vi "Autonomous Independent.vi"() -> ()   [LabVIEW 2017]
doc: "This VI is called when autonomous begins, and will automatically be terminated when autonomous ends. You can carry out timed or sensor driven robot movement independently without needing to return to the caller."
uses:
  Public/Documents/Cross The Road Electronics/Phoenix-LabVIEW/Motor Controller/Controls/CTRE_Phoenix_MotorControl_ControlMode.ctl
  <vilib>/Rock Robotics/WPI/DriverStation/WPI_DriverStationAllianceInfo.ctl
  <vilib>/Rock Robotics/WPI/Relay/WPI_RelayValue.ctl
  <vilib>/Rock Robotics/WPI/SerialPort/WPI_SerialPort.ctl
  <vilib>/Rock Robotics/WPI/Utilities/WPI_GetSetVariantRefNum.vi
  Public/Documents/Cross The Road Electronics/Phoenix-LabVIEW/Motor Controller/Get/CTRE_Phoenix_MotorController_GetPulseWidthAll.vi
  Robot Global Data.vi
  <vilib>/Utility/config.llb/Read Key (Double).vi
  Public/Documents/Cross The Road Electronics/Phoenix-LabVIEW/Motor Controller/Get/CTRE_Phoenix_MotorController_GetSelectedSensorData.vi
  Public/Documents/Cross The Road Electronics/Phoenix-LabVIEW/Motor Controller/Get/CTRE_Phoenix_MotorController_GetQuadratureData.vi
  <vilib>/Rock Robotics/WPI/Solenoid/Deprecated/WPI_SolenoidSetBool.vi
  <vilib>/Utility/config.llb/NI_LVConfig.lvlib
panel:
  out "Current Pos 3":dbl
  out "Current Pos 2":dbl
  out "Current Pos 1":dbl
  out "Current Pos 0":dbl
  out "ElevatorScale":dbl
  out "ElevatorSwitch":dbl
  out "ElevatorPyramid":dbl
  out "ElevatorDown":dbl
  out "ElevatePos":dbl
  out "CoolDown":bool
  out "MidSwitchPosition":dbl
  out "zChange":dbl
  out "Gyro":dbl
  out "Zero Gyro":bool
  out "Autonomous Select":dbl
  out "Direction":dbl
  out "stopped":bool
  out "speed":dbl
  out "Direction 3":dbl
  out "Direction 2":dbl
  out "Direction 1":dbl
  out "x":dbl
  out "Current Reading":string
  out "Text":string
  out "Switch":bool
  out "Scale":bool
  out "Rel Pos 3":i32
  out "Rel Pos 2":i32
  out "Rel Pos 1":i32
  out "Rel Pos 0":i32
  out "Final Rel Pos 3":i32
  out "Final Rel Pos 2":i32
  out "Final Rel Pos 1":i32
  out "Final Rel Pos 0":i32
  out "Start Pos 3":i32
  out "Start Pos 2":i32
  out "Start Pos 1":i32
  out "Start Pos 0":i32
  # "Be sure to right-click and choose Data Operations>>Make Current Value default if you want to save the array values with the VI"
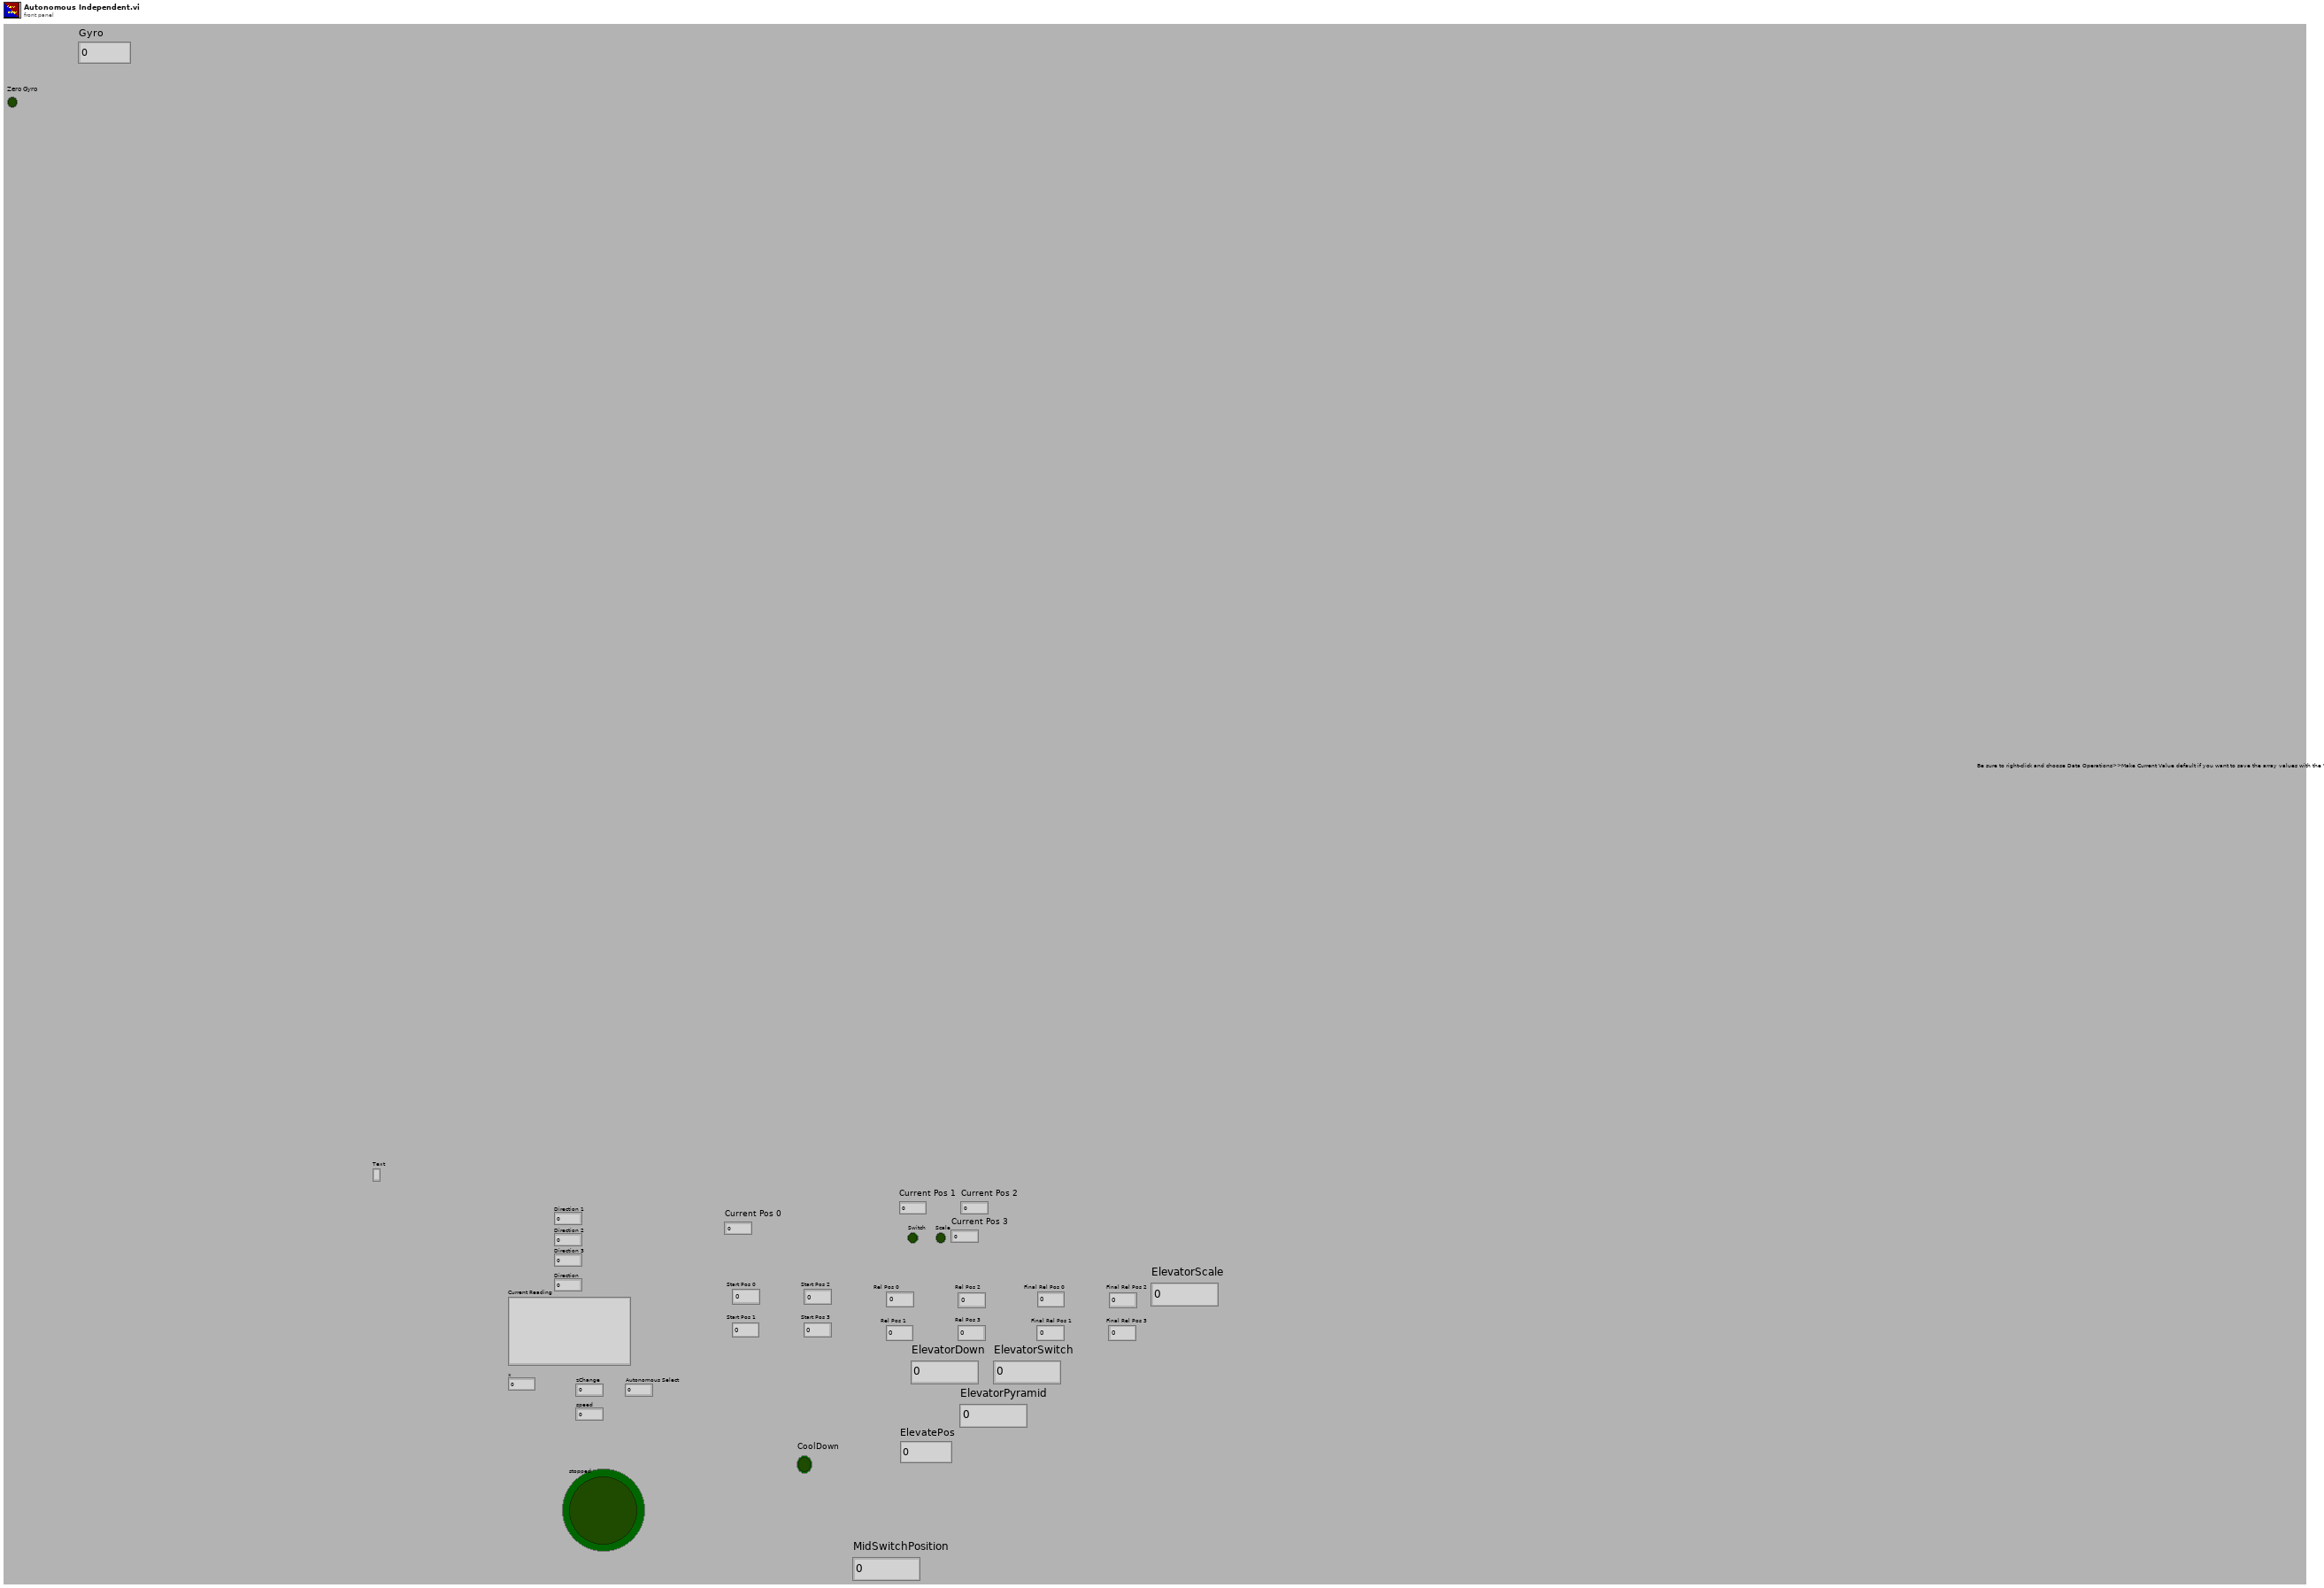
[diagram p1: front panel]
types:
  T1 = typedef "WPI_JoystickDevRef.ctl" = cluster{"Device":T2}
  T2 = typedef "WPI_JoystickDeviceEnum.ctl" = enum16{"USB 0", "USB 1", "USB 2", "USB 3", "USB 4", "USB 5"}
  T3 = typedef "WPI_DriverStationAllianceInfo.ctl" = enum16{"Red", "Blue", "Invalid"}
  T4 = typedef "WPI_RelayValue.ctl" = enum16{"Off", "On", "Forward", "Reverse"}
  T5 = typedef "WPI_SerialPort.ctl" = enum16{"Onboard RS-232", "MXP TTL", "USB 1", "USB 2"}
  T6 = typedef "CTRE_Phoenix_MotorControl_ControlMode.ctl" = u16
  T7 = typedef "WPI_GyroDevRef.ctl" = cluster{"DevStatus":errorcluster, "Analog Channel":T8, "Gain (VoltsPerDegree/Second)":dbl, "Gyro Type":enum16{"Analog", "XRS450"}, "Handle":i32, "SPI Bus":T9, "Device Found":bool, "Sample Rate":dbl, "Calibrate On Open":bool, "Offset":dbl}
  T8 = typedef "FPGA_AIChannel.ctl" = enum8{"AI 0", "AI 1", "AI 2", "AI 3", "AI MXP 0", "AI MXP 1", "AI MXP 2", "AI MXP 3", "Invalid"}
  T9 = typedef "spi_bus.ctl" = enum16{"SPI On-Board, CS0", "SPI On-Board, CS1", "SPI On-Board, CS2", "SPI On-Board, CS3", "SPI MXP", "Invalid"}
  T10 = typedef "WPI_MotorControlDeviceRef.ctl" = cluster{"DeviceStatus":errorcluster, "Type":T11, "PWM":cluster{"PWM Channel":T12, "DeadBand":T13}, "CAN":cluster{"Device Number":u8, "SetOutput VI Ref":variant, "GetOutput VI Ref":variant, "Enable VI Ref":variant, "Disable VI Ref":variant, "Data":variant}, "Invert":bool, "DIO PWM":cluster{"PWM \"Enable\" Channel":T12, "DIOChannel":T14, "PWM Rate":dbl}}
  T11 = typedef "WPI_MotorControlType.ctl" = enum16{"PWM", "CAN", "DIO PWM"}
  T12 = typedef "FPGA_DIOPWMChannel.ctl" = enum8{"PWM 0", "PWM 1", "PWM 2", "PWM 3", "PWM 4", "PWM 5", "PWM 6", "PWM 7", "PWM 8", "PWM 9", "PWM MXP 0", "PWM MXP 1", "PWM MXP 2", "PWM MXP 3", "PWM MXP 4", "PWM MXP 5", "PWM MXP 6", "PWM MXP 7", "PWM MXP 8", "PWM MXP 9", "Invalid"}
  T13 = typedef "WPI_PWMDeadband.ctl" = cluster{"Name":string, "maxPositivePwm":i32, "minPositivePwm":i32, "centerPwm":i32, "maxNegativePwm":i32, "minNegativePwm":i32, "angularRange":u16}
  T14 = typedef "FPGA_DIOChannel.ctl" = enum8{"DIO 0", "DIO 1", "DIO 2", "DIO 3", "DIO 4", "DIO 5", "DIO 6", "DIO 7", "DIO 8", "DIO 9", "DIO MXP 0", "DIO MXP 1", "DIO MXP 2", "DIO MXP 3", "DIO MXP 4", "DIO MXP 5", "DIO MXP 6", "DIO MXP 7", "DIO MXP 8", "DIO MXP 9", "DIO MXP 10", "DIO MXP 11", "DIO MXP 12", "DIO MXP 13", "DIO MXP 14", "DIO MXP 15", "SPI Port CS1", "SPI Port CS2", "SPI Port CS3", "SPI Port MISO", "SPI Port MOSI", "Invalid"}
  T15 = typedef "NI_LVConfig.lvlib/Config Data RefNum.ctl" = refnum<k1>
  T16 = typedef "WPI_RelayDevRef.ctl" = cluster{"DevStatus":errorcluster, "Relay Channel":T17, "Relay Direction":T18}
  T17 = typedef "FPGA_DIORelayChannel.ctl" = enum8{"Relay 0", "Relay 1", "Relay 2", "Relay 3", "Invalid"}
  T18 = typedef "WPI_RelayDirection.ctl" = enum16{"Both directions", "Forward only", "Reverse only"}
  T19 = typedef "WPI_SerialPortRef.ctl" = cluster{"DevStatus":errorcluster, "Serial Port Name":refnum<visa-resource-name>}
  T20 = typedef "WPI_SolenoidDevRef.ctl" = cluster{"DevStatus":errorcluster, "Pneumatics Control Module":u8, "Forward Solenoid Channel":T21, "Reverse Solenoid Channel":T21}
  T21 = typedef "WPI_SolenoidChannel.ctl" = enum8{"Solenoid 0", "Solenoid 1", "Solenoid 2", "Solenoid 3", "Solenoid 4", "Solenoid 5", "Solenoid 6", "Solenoid 7", "Invalid"}
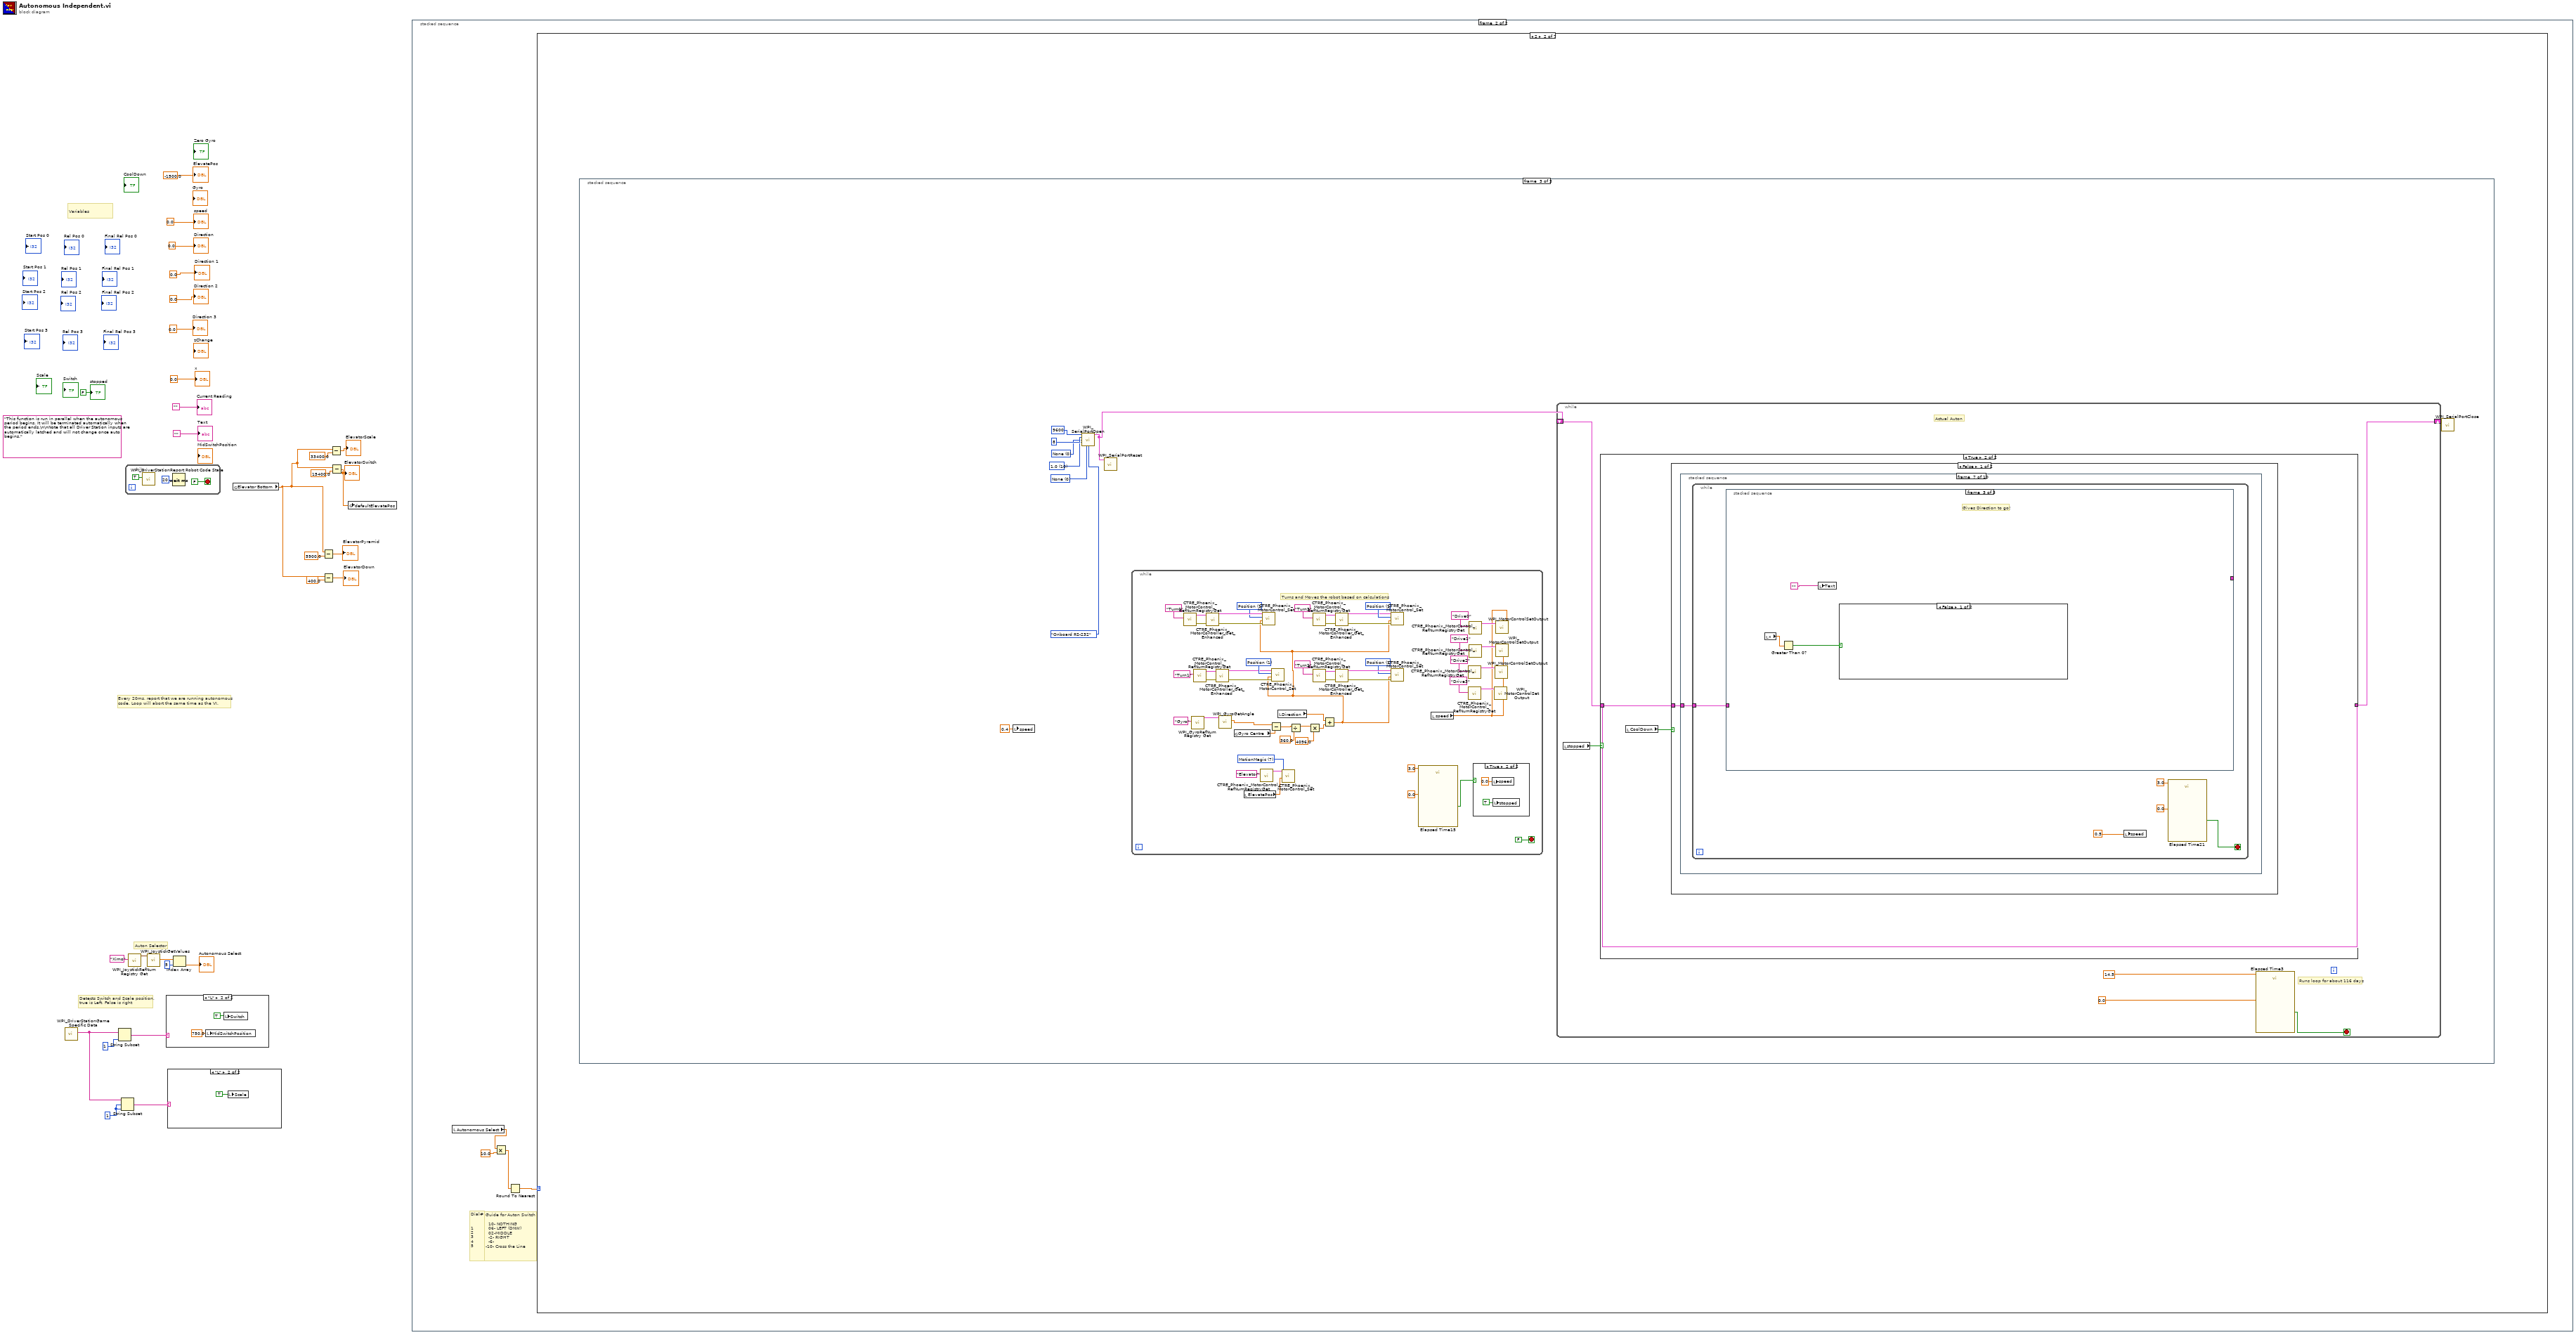
[diagram p0: block diagram]
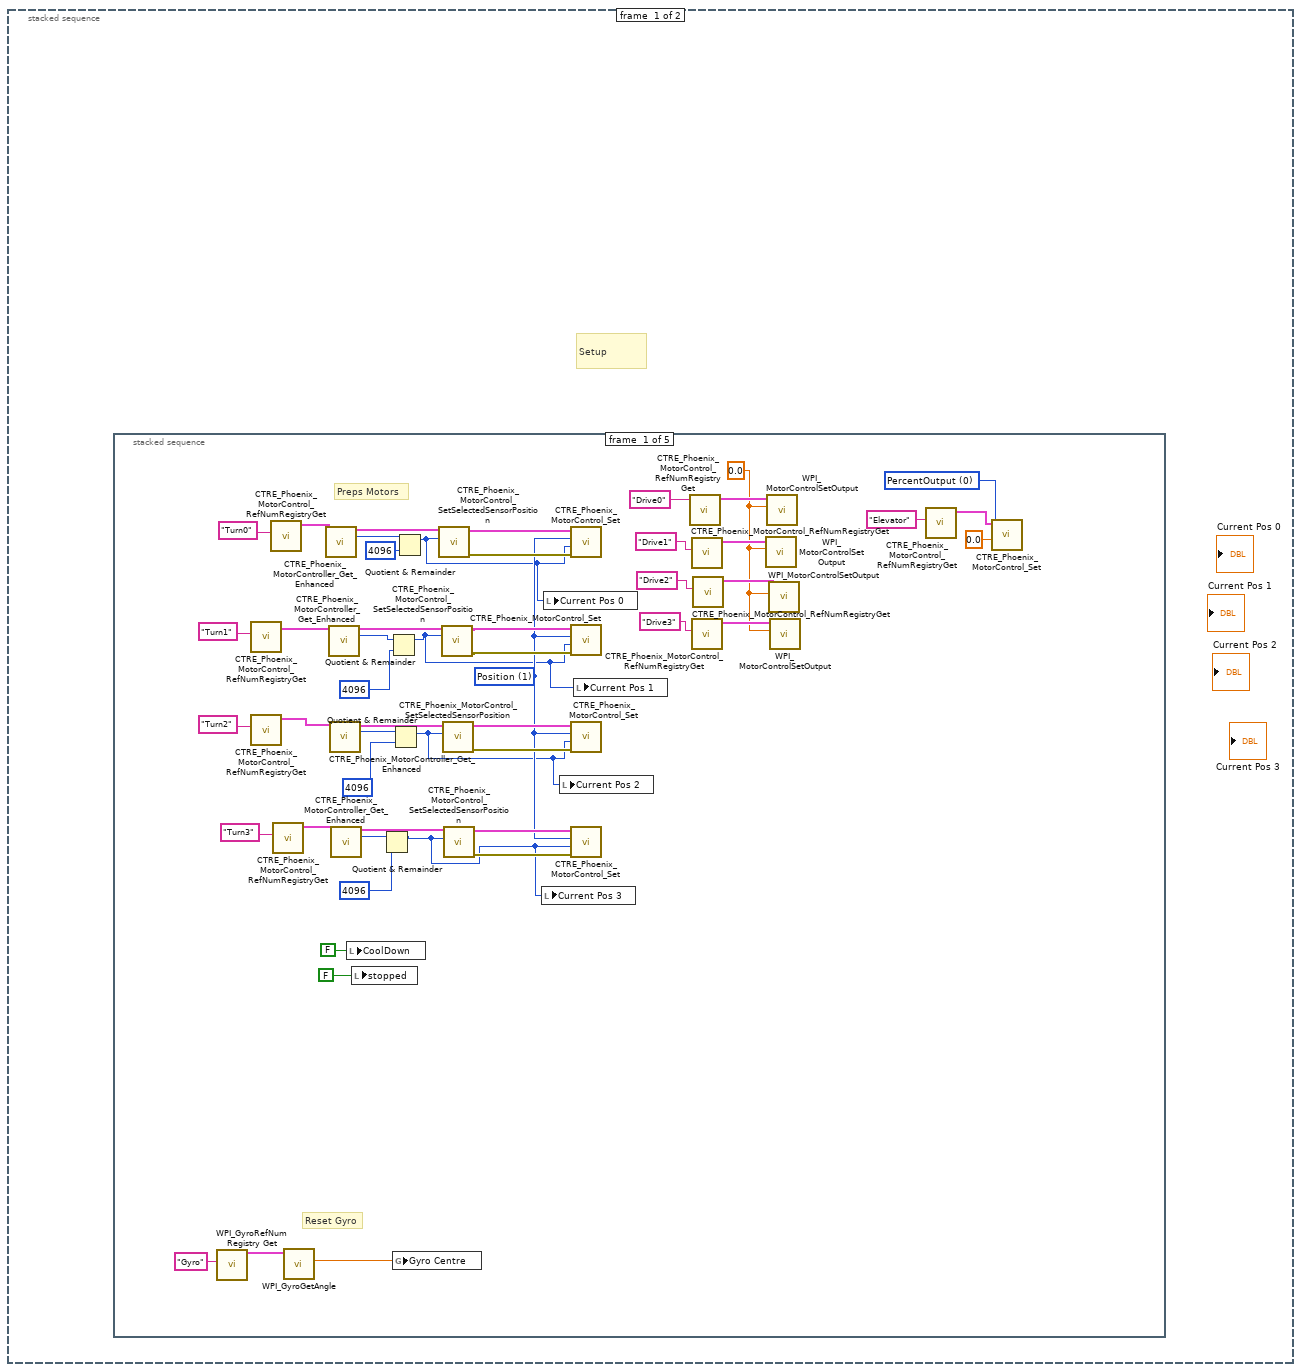
[diagram p2: hidden frame]
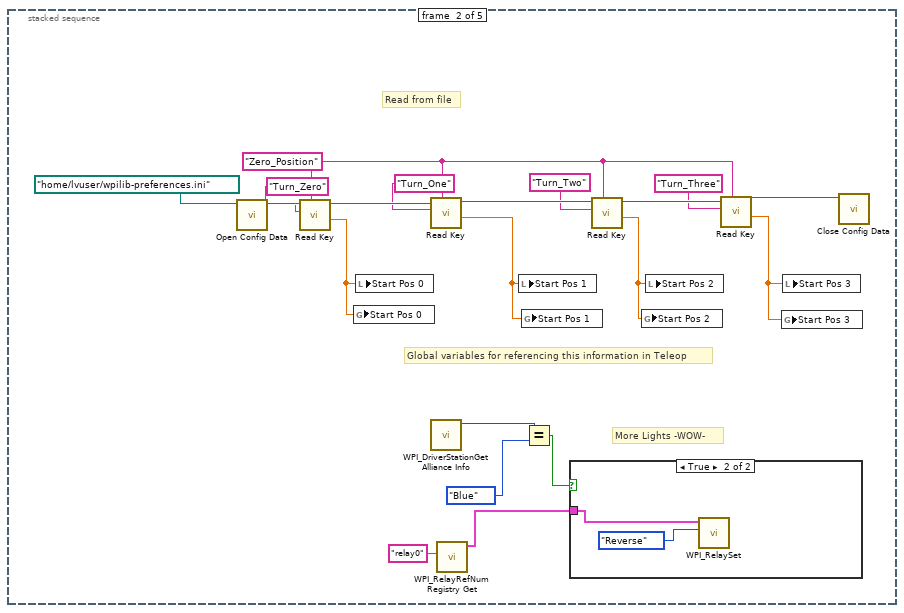
[diagram p3: hidden frame]
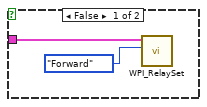
[diagram p4: hidden frame]
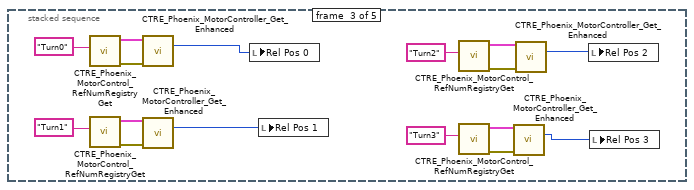
[diagram p5: hidden frame]
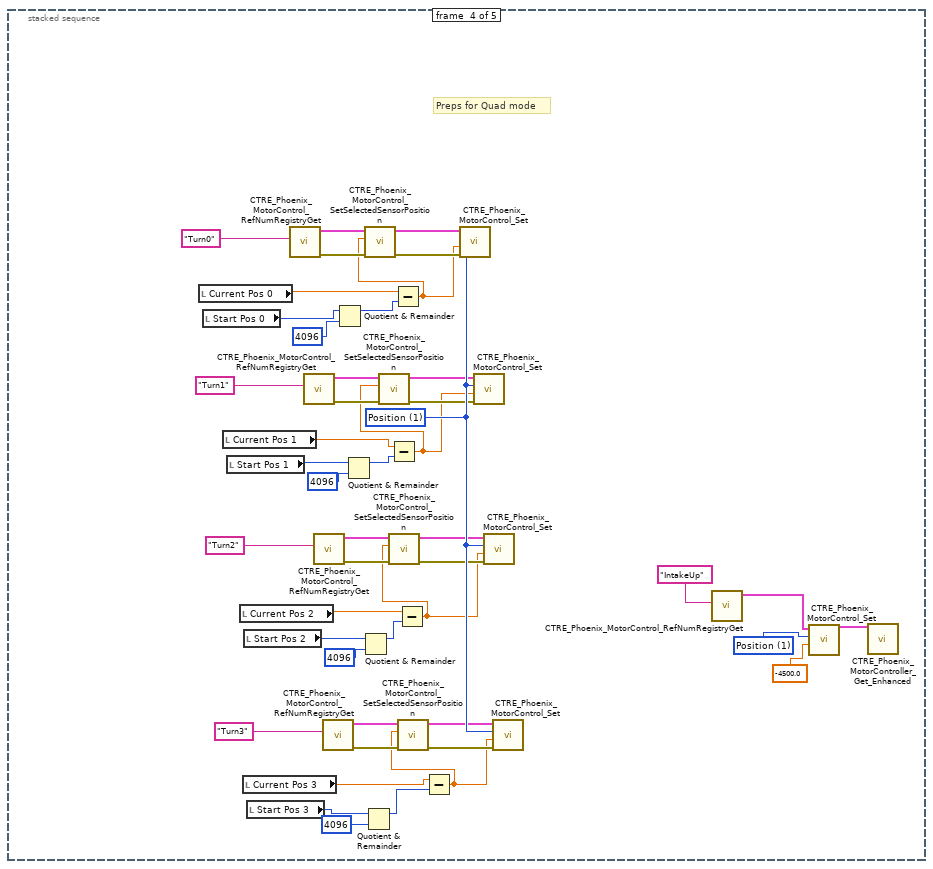
[diagram p6: hidden frame]
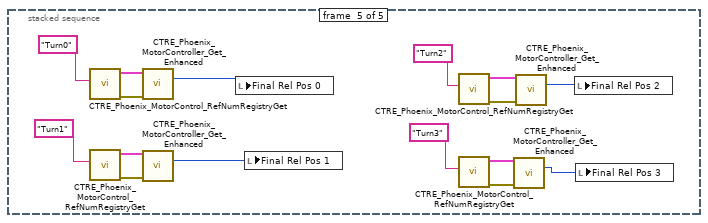
[diagram p7: hidden frame]
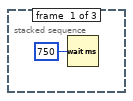
[diagram p9: hidden frame]
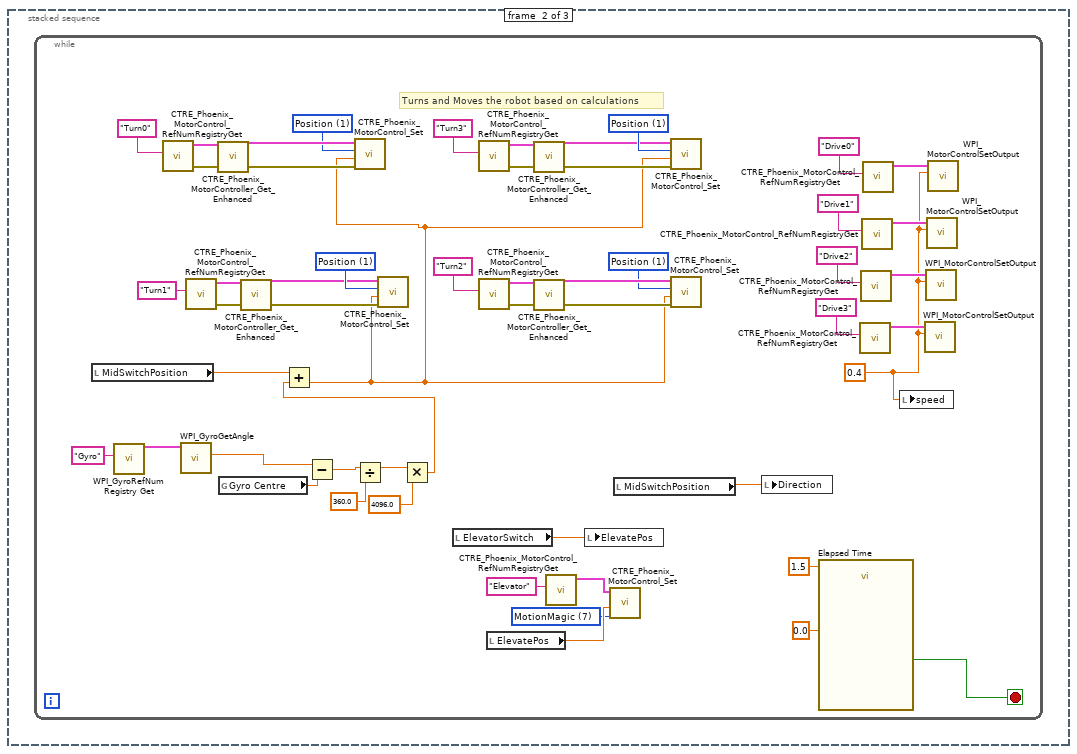
[diagram p10: hidden frame]
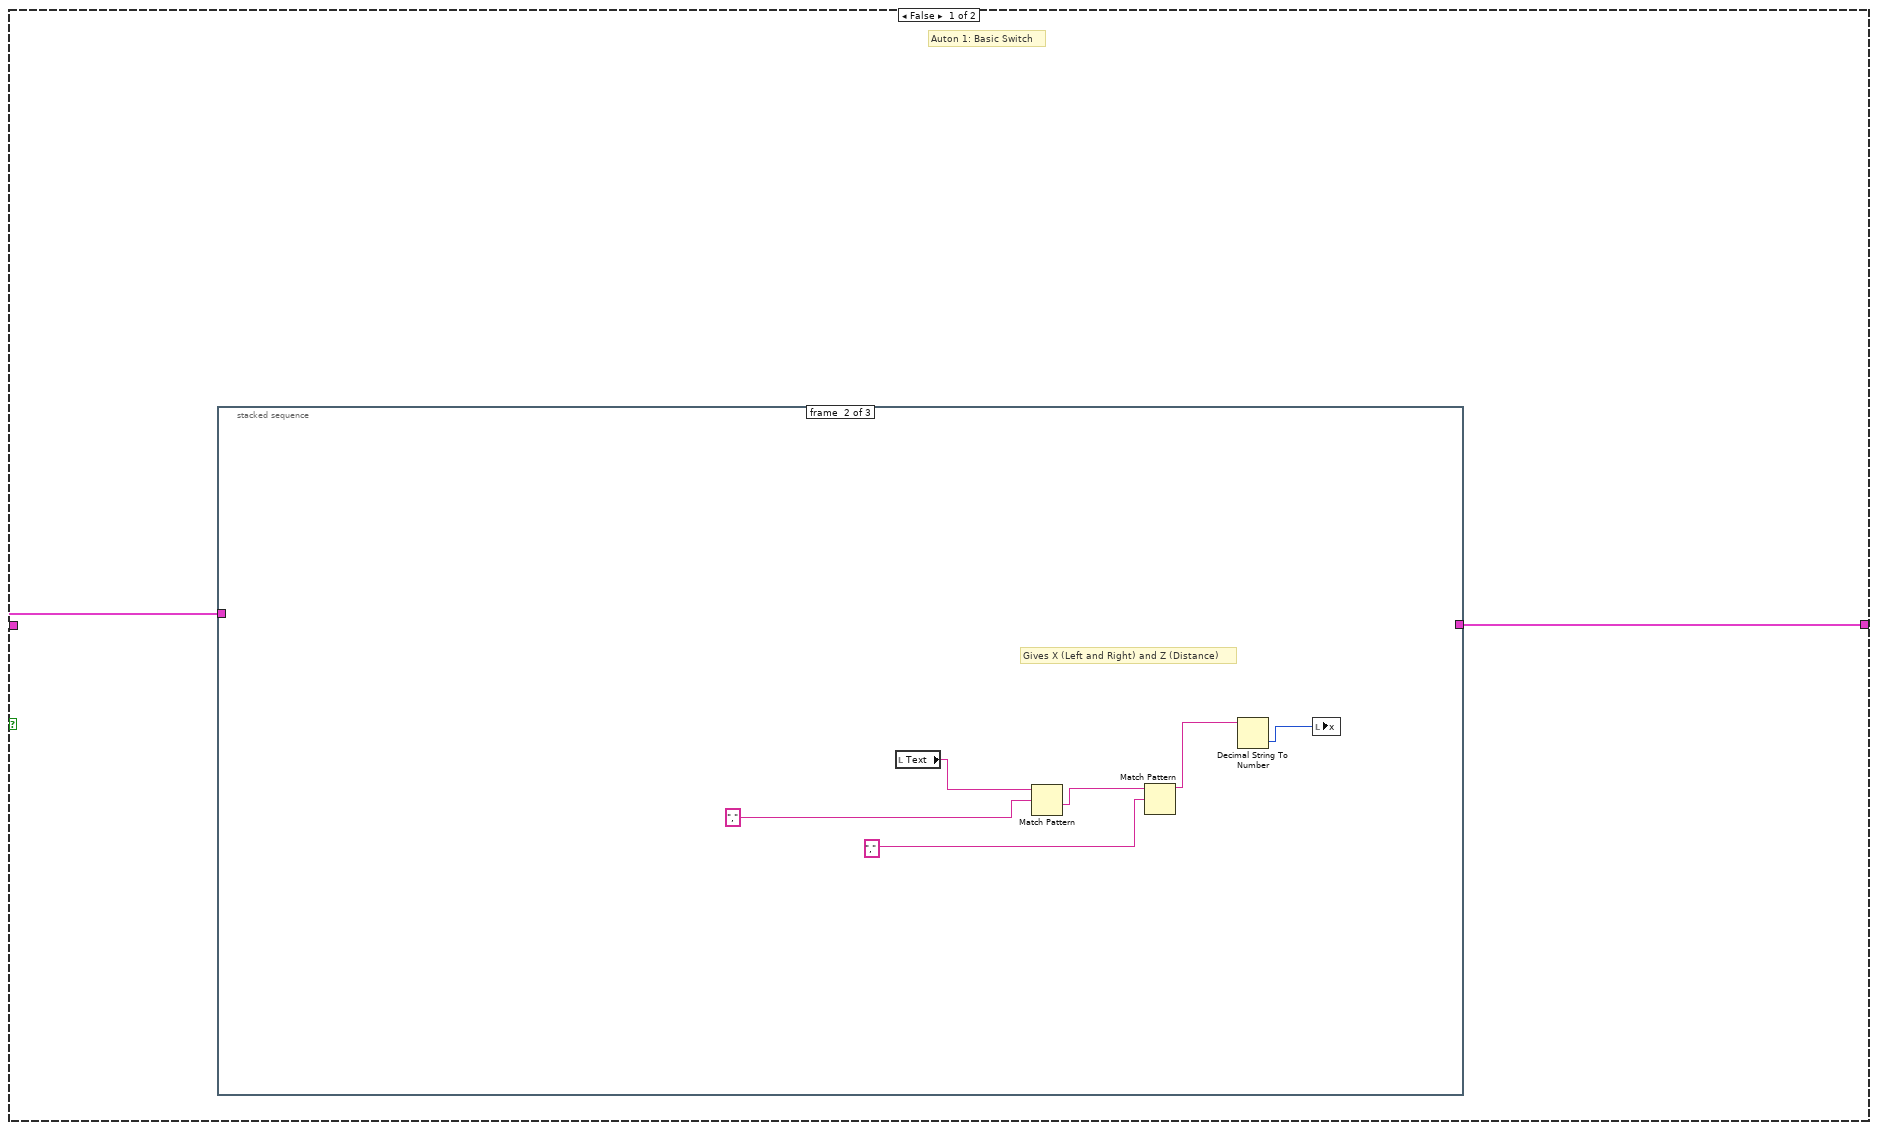
[diagram p12: hidden frame]
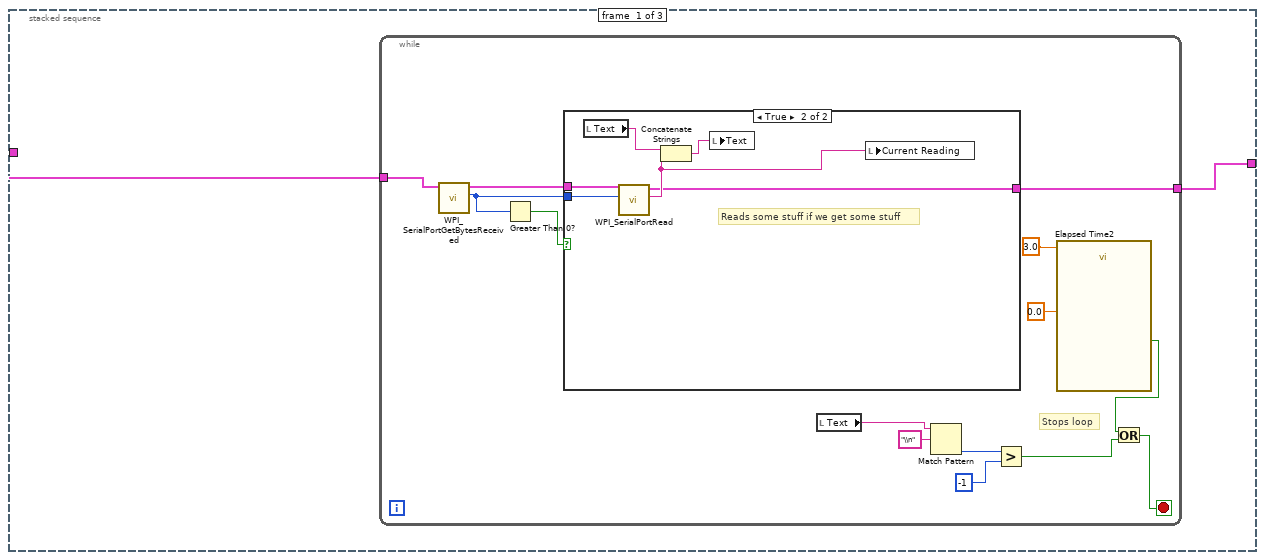
[diagram p13: hidden frame]
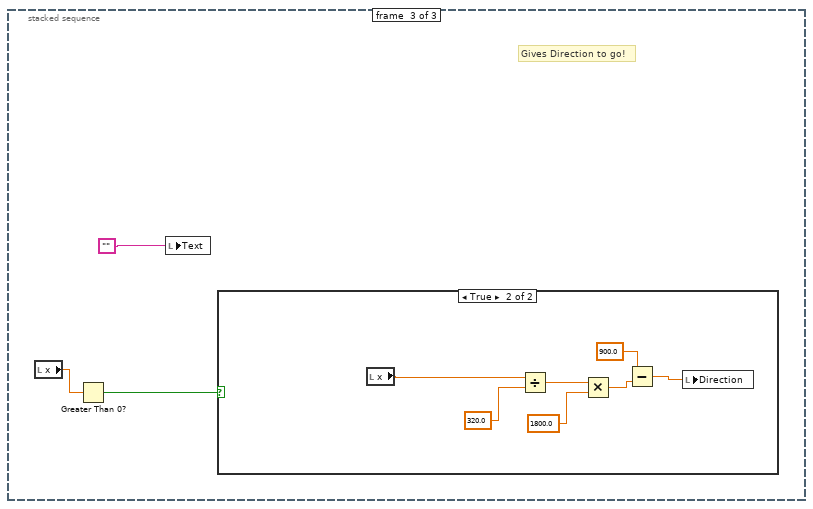
[diagram p15: hidden frame]
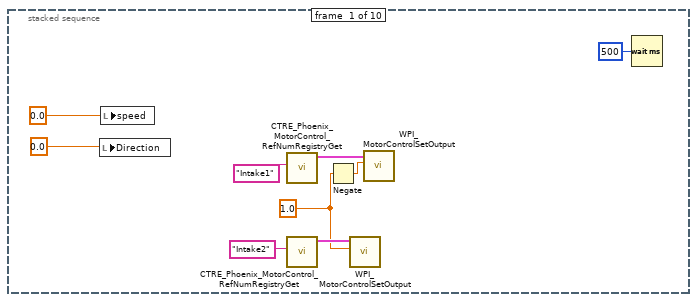
[diagram p17: hidden frame]
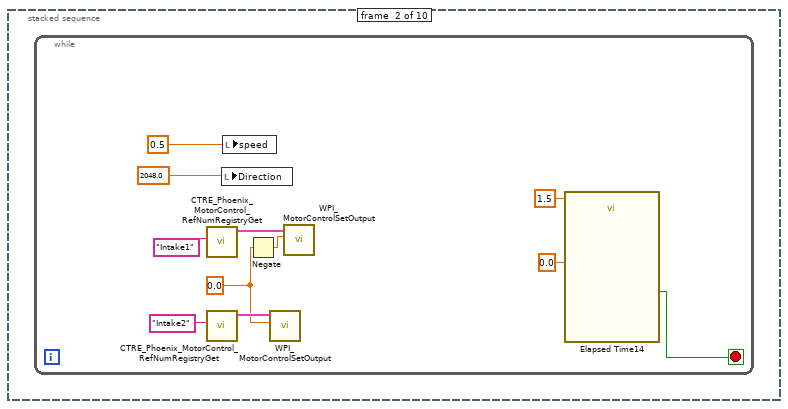
[diagram p18: hidden frame]
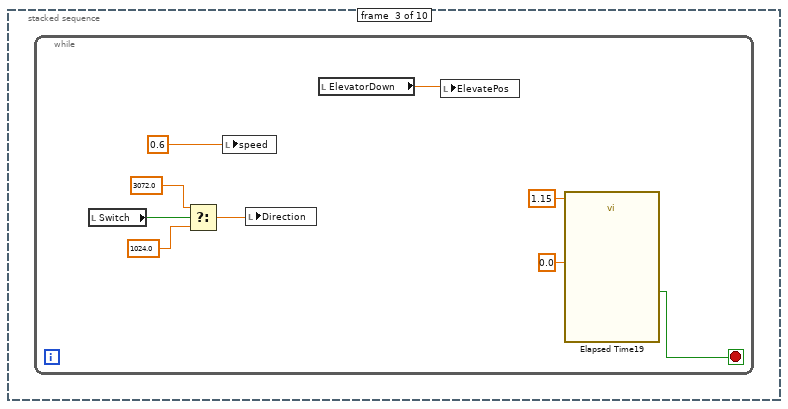
[diagram p19: hidden frame]
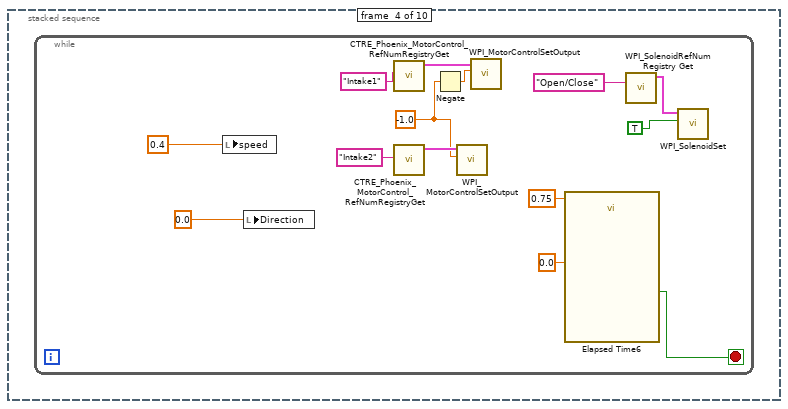
[diagram p20: hidden frame]
diagram:
  w26 = 1 ("length (rest)")
  (unwired) "This function is run in parallel when the autonomous period begins. It will be terminated automatically when the period ends.\n\nNote that all Driver Station inputs are automatically latched and will not change once auto begins."
  # "Auton Selector"
  # "Variables"
  # "Detects Switch and Scale position,\ntrue is Left, False is right"
  # "Every 20ms, report that we are running autonomous\ncode. Loop will abort the same time as the VI."
  n1 = call <vilib>:"WPI_DriverStationGame Specific Data.vi"() -> ("Game Specific Data"=w25:string)  [unwired: 11 in]
  n2 = String Subset(string=w25, length (rest)=1 ("length (rest)")) -> (substring=w29:string)  [unwired: 1 in]
  n3 = String Subset(string=w25, offset (0)=w26, length (rest)=w26) -> (substring=w27:string)
  n4 = while {
    stop <- FALSE stop-if-true
    n5 = call <vilib>:"WPI_DriverStationReport Robot Code State.vi"("Autonomous"=TRUE) -> ()  [unwired: 10 in, 1 out]
    n6 = Wait (ms)(milliseconds to wait=u32 20) -> ()  [unwired: 1 out]
  }
  n7 = call <vilib>:"WPI_JoystickRefNum Registry Get.vi"("refnum name"="Ximo") -> ("JoystickDevRef"=w23:T1)  [unwired: 9 in, 1 out]
  n8 = call <vilib>:"WPI_JoystickGetValues.vi"("JoystickDevRef"=w23) -> ("Axes"=w22:dbl[])  [unwired: 6 in, 4 out]
  n9 = case shown="\"L\"" w29 {
    frame "R", Default {
      n10 = local write "MidSwitchPosition"(-750.0 ("MidSwitchPosition")) -> ()
      n11 = local write "Switch"(FALSE ("Switch")) -> ()
    }
    frame "L" {
      n12 = local write "MidSwitchPosition"(750.0 ("MidSwitchPosition")) -> ()
      n13 = local write "Switch"(TRUE ("Switch")) -> ()
    }
  }
  n14 = case shown="\"L\"" w27 {
    frame "R", Default {
      n15 = local write "Scale"(FALSE ("Switch")) -> ()
    }
    frame "L" {
      n16 = local write "Scale"(TRUE ("Switch")) -> ()
    }
  }
  n17 = Index Array(array=w22, index=5) -> (element=→"Autonomous Select":dbl)
  n18 = global read "Robot Global Data.vi" "Elevator Bottom"() -> (w4:dbl)
  n19 = Subtract(x=w4, y=5900.0) -> (x-y=→"ElevatorPyramid":dbl)
  n20 = Subtract(x=w4, y=400.0) -> (x-y=→"ElevatorDown":dbl)
  n21 = Subtract(x=w4, y=33400.0 ("ElevatorScale")) -> (x-y=→"ElevatorScale":dbl)
  n22 = Subtract(x=w4, y=15400.0 ("ElevatorSwitch")) -> (x-y=w1:dbl)
  "ElevatorSwitch" <- w1
  n23 = global write "Robot Global Data.vi" "defaultElevatePos"(w1) -> ()
  n24 = stacked-sequence {
    frame #0 {
      # "Setup"
      n25 = stacked-sequence {
        frame #0 {
          w45 = T6 0 items=["PercentOutput"=0, "Position"=1, "Velocity"=2, "Current"=3, "Follower"=5, "MotionProfile"=6, "MotionMagic"=7, "MotionMagicArc"=8, "MotionProfileArc"=10, "Disabled"=15] ("Control Mode")
          w54 = 0.0 ("Output")
          w43 = T6 1 items=["PercentOutput"=0, "Position"=1, "Velocity"=2, "Current"=3, "Follower"=5, "MotionProfile"=6, "MotionMagic"=7, "MotionMagicArc"=8, "MotionProfileArc"=10, "Disabled"=15] ("Control Mode")
          # "Reset Gyro"
          # "Preps Motors"
          n26 = call <vilib>:"WPI_GyroRefNum Registry Get.vi"("refnum name"="Gyro") -> ("GyroDevRef"=w61:T7)  [unwired: 9 in, 1 out]
          n27 = call "CTRE_Phoenix_MotorControl_RefNumRegistryGet.vi"("refnum name"="Turn1") -> ("PhoenixMotorControlDevRef"=w69:T10)  [unwired: 9 in, 1 out]
          n28 = call "CTRE_Phoenix_MotorControl_RefNumRegistryGet.vi"("refnum name"="Turn2") -> ("PhoenixMotorControlDevRef"=w68:T10)  [unwired: 9 in, 1 out]
          n29 = call "CTRE_Phoenix_MotorControl_RefNumRegistryGet.vi"("refnum name"="Turn0") -> ("PhoenixMotorControlDevRef"=w70:T10)  [unwired: 9 in, 1 out]
          n30 = call "CTRE_Phoenix_MotorControl_RefNumRegistryGet.vi"("refnum name"="Turn3") -> ("PhoenixMotorControlDevRef"=w67:T10)  [unwired: 9 in, 1 out]
          n31 = call <vilib>:"WPI_GyroGetAngle.vi"("GyroDevRef"=w61) -> ("Angle"=w50:dbl)  [unwired: 6 in, 4 out]
          n32 = call-poly "CTRE_Phoenix_MotorController_Get_Enhanced.vi"("PhoenixMotorControlDevRef"=w70) -> ("PhoenixMotorControlDevRef"=w89:T10, "Pulse Width Position"=w77:i32)  [unwired: 9 in, 4 out]
          n33 = call-poly "CTRE_Phoenix_MotorController_Get_Enhanced.vi"("PhoenixMotorControlDevRef"=w69) -> ("PhoenixMotorControlDevRef"=w88:T10, "Pulse Width Position"=w65:i32)  [unwired: 9 in, 4 out]
          n34 = call-poly "CTRE_Phoenix_MotorController_Get_Enhanced.vi"("PhoenixMotorControlDevRef"=w68) -> ("PhoenixMotorControlDevRef"=w87:T10, "Pulse Width Position"=w76:i32)  [unwired: 9 in, 4 out]
          n35 = call-poly "CTRE_Phoenix_MotorController_Get_Enhanced.vi"("PhoenixMotorControlDevRef"=w67) -> ("PhoenixMotorControlDevRef"=w86:T10, "Pulse Width Position"=w75:i32)  [unwired: 9 in, 4 out]
          n36 = local write "CoolDown"(FALSE ("Switch")) -> ()
          n37 = local write "stopped"(FALSE ("Switch")) -> ()
          n38 = Quotient & Remainder(x=w75, y=4096) -> (x-y*floor(x/y)=w42:i32)  [unwired: 1 out]
          n39 = Quotient & Remainder(x=w65, y=4096) -> (x-y*floor(x/y)=w40:i32)  [unwired: 1 out]
          n40 = Quotient & Remainder(x=w76, y=4096) -> (x-y*floor(x/y)=w41:i32)  [unwired: 1 out]
          n41 = global write "Robot Global Data.vi" "Gyro Centre"(w50) -> ()
          n42 = Quotient & Remainder(x=w77, y=4096) -> (x-y*floor(x/y)=w39:i32)  [unwired: 1 out]
          n43 = call "CTRE_Phoenix_MotorControl_SetSelectedSensorPosition.vi"("New Sensor Position"=w39, "PhoenixMotorControlDevRef"=w89) -> ("error out"=w84:errorcluster, "PhoenixMotorControlDevRef"=w85:T10)  [unwired: 8 in]
          n44 = call "CTRE_Phoenix_MotorControl_SetSelectedSensorPosition.vi"("New Sensor Position"=w40, "PhoenixMotorControlDevRef"=w88) -> ("error out"=w82:errorcluster, "PhoenixMotorControlDevRef"=w83:T10)  [unwired: 8 in]
          n45 = call "CTRE_Phoenix_MotorControl_SetSelectedSensorPosition.vi"("New Sensor Position"=w41, "PhoenixMotorControlDevRef"=w87) -> ("error out"=w80:errorcluster, "PhoenixMotorControlDevRef"=w81:T10)  [unwired: 8 in]
          n46 = call "CTRE_Phoenix_MotorControl_SetSelectedSensorPosition.vi"("New Sensor Position"=w42, "PhoenixMotorControlDevRef"=w86) -> ("error out"=w78:errorcluster, "PhoenixMotorControlDevRef"=w79:T10)  [unwired: 8 in]
          n47 = local write "Current Pos 3"(w42) -> ()
          n48 = local write "Current Pos 0"(w39) -> ()
          n49 = local write "Current Pos 2"(w41) -> ()
          n50 = call "CTRE_Phoenix_MotorControl_Set.vi"("error in (no error)"=w84, "Output"=w39, "Control Mode"=w43, "PhoenixMotorControlDevRef"=w85) -> ()  [unwired: 6 in, 2 out]
          n51 = call "CTRE_Phoenix_MotorControl_Set.vi"("error in (no error)"=w82, "Output"=w40, "Control Mode"=w43, "PhoenixMotorControlDevRef"=w83) -> ()  [unwired: 6 in, 2 out]
          n52 = call "CTRE_Phoenix_MotorControl_Set.vi"("error in (no error)"=w80, "Output"=w41, "Control Mode"=w43, "PhoenixMotorControlDevRef"=w81) -> ()  [unwired: 6 in, 2 out]
          n53 = call "CTRE_Phoenix_MotorControl_Set.vi"("error in (no error)"=w78, "Output"=w42, "Control Mode"=w43, "PhoenixMotorControlDevRef"=w79) -> ()  [unwired: 6 in, 2 out]
          n54 = local write "Current Pos 1"(w40) -> ()
          n55 = call "CTRE_Phoenix_MotorControl_RefNumRegistryGet.vi"("refnum name"="Drive0") -> ("PhoenixMotorControlDevRef"=w56:T10)  [unwired: 9 in, 1 out]
          n56 = call "CTRE_Phoenix_MotorControl_RefNumRegistryGet.vi"("refnum name"="Drive1") -> ("PhoenixMotorControlDevRef"=w57:T10)  [unwired: 9 in, 1 out]
          n57 = call "CTRE_Phoenix_MotorControl_RefNumRegistryGet.vi"("refnum name"="Drive3") -> ("PhoenixMotorControlDevRef"=w58:T10)  [unwired: 9 in, 1 out]
          n58 = call "CTRE_Phoenix_MotorControl_RefNumRegistryGet.vi"("refnum name"="Drive2") -> ("PhoenixMotorControlDevRef"=w55:T10)  [unwired: 9 in, 1 out]
          n59 = call <vilib>:"WPI_MotorControlSetOutput.vi"("Output"=w54, "MotorControlDevRef"=w57) -> ()  [unwired: 7 in, 3 out]
          n60 = call <vilib>:"WPI_MotorControlSetOutput.vi"("Output"=w54, "MotorControlDevRef"=w56) -> ()  [unwired: 7 in, 3 out]
          n61 = call <vilib>:"WPI_MotorControlSetOutput.vi"("Output"=w54, "MotorControlDevRef"=w55) -> ()  [unwired: 7 in, 3 out]
          n62 = call <vilib>:"WPI_MotorControlSetOutput.vi"("Output"=w54, "MotorControlDevRef"=w58) -> ()  [unwired: 7 in, 3 out]
          n63 = call "CTRE_Phoenix_MotorControl_RefNumRegistryGet.vi"("refnum name"="Elevator") -> ("PhoenixMotorControlDevRef"=w46:T10)  [unwired: 9 in, 1 out]
          n64 = call "CTRE_Phoenix_MotorControl_Set.vi"("Output"=0.0, "Control Mode"=w45, "PhoenixMotorControlDevRef"=w46) -> ()  [unwired: 7 in, 2 out]
        }
        frame #1 {
          w99 = "Zero_Position" ("section")
          # "More Lights -WOW-"
          # "Global variables for referencing this information in Teleop"
          # "Read from file"
          n65 = call <vilib>:"Open Config Data.vi"("configuration file path"=path "/home/lvuser/wpilib-preferences.ini") -> ("refnum"=w109:T15)  [unwired: 8 in, 2 out]
          n66 = call-poly <vilib>:"Read Key.vi"("section"=w99, "key"="Turn_Zero", "refnum"=w109) -> ("value"=w98:dbl, "refnum out"=w108:T15)  [unwired: 5 in, 2 out]
          n67 = global write "Robot Global Data.vi" "Start Pos 0"(w98) -> ()
          n68 = local write "Start Pos 0"(w98) -> ()
          n69 = call-poly <vilib>:"Read Key.vi"("section"=w99, "key"="Turn_One", "refnum"=w108) -> ("value"=w97:dbl, "refnum out"=w107:T15)  [unwired: 5 in, 2 out]
          n70 = call <vilib>:"WPI_DriverStationGet Alliance Info.vi"() -> ("Alliance"=w94:T3)  [unwired: 11 out]
          n71 = call <vilib>:"WPI_RelayRefNum Registry Get.vi"("refnum name"="relay0") -> ("RelayDevRef"=w92:T16)  [unwired: 9 in, 1 out]
          n72 = local write "Start Pos 1"(w97) -> ()
          n73 = global write "Robot Global Data.vi" "Start Pos 1"(w97) -> ()
          n74 = Equal?(x=w94, y=WPI_DriverStationAllianceInfo."Blue" ("Alliance")) -> (x = y?=w93:bool)
          n75 = case shown="True" w93 {
            tunnel: w92 -> [w110 w112]
            frame False {
              n76 = call <vilib>:"WPI_RelaySet.vi"("RelayValue"=WPI_RelayValue."Forward", "RelayDevRef"=w110) -> ()  [unwired: 8 in, 2 out]
            }
            frame True {
              n77 = call <vilib>:"WPI_RelaySet.vi"("RelayValue"=WPI_RelayValue."Reverse", "RelayDevRef"=w112) -> ()  [unwired: 8 in, 2 out]
            }
          }
          n78 = call-poly <vilib>:"Read Key.vi"("section"=w99, "key"="Turn_Two", "refnum"=w107) -> ("value"=w96:dbl, "refnum out"=w106:T15)  [unwired: 5 in, 2 out]
          n79 = global write "Robot Global Data.vi" "Start Pos 2"(w96) -> ()
          n80 = local write "Start Pos 2"(w96) -> ()
          n81 = call-poly <vilib>:"Read Key.vi"("section"=w99, "key"="Turn_Three", "refnum"=w106) -> ("value"=w95:dbl, "refnum out"=w105:T15)  [unwired: 5 in, 2 out]
          n82 = global write "Robot Global Data.vi" "Start Pos 3"(w95) -> ()
          n83 = local write "Start Pos 3"(w95) -> ()
          n84 = call <vilib>:"Close Config Data.vi"("refnum"=w105) -> ()  [unwired: 9 in, 2 out]
        }
        frame #2 {
          n85 = call "CTRE_Phoenix_MotorControl_RefNumRegistryGet.vi"("refnum name"="Turn0") -> ("error out"=w124:errorcluster, "PhoenixMotorControlDevRef"=w125:T10)  [unwired: 9 in]
          n86 = call "CTRE_Phoenix_MotorControl_RefNumRegistryGet.vi"("refnum name"="Turn1") -> ("error out"=w122:errorcluster, "PhoenixMotorControlDevRef"=w123:T10)  [unwired: 9 in]
          n87 = call-poly "CTRE_Phoenix_MotorController_Get_Enhanced.vi"("PhoenixMotorControlDevRef"=w125, "error in"=w124) -> ("Position (Raw Sensor Units)"=w117:i32)  [unwired: 10 in, 3 out]
          n88 = call-poly "CTRE_Phoenix_MotorController_Get_Enhanced.vi"("PhoenixMotorControlDevRef"=w123, "error in"=w122) -> ("Position (Raw Sensor Units)"=w116:i32)  [unwired: 10 in, 3 out]
          n89 = local write "Rel Pos 0"(w117) -> ()
          n90 = local write "Rel Pos 1"(w116) -> ()
          n91 = call "CTRE_Phoenix_MotorControl_RefNumRegistryGet.vi"("refnum name"="Turn2") -> ("error out"=w120:errorcluster, "PhoenixMotorControlDevRef"=w121:T10)  [unwired: 9 in]
          n92 = call "CTRE_Phoenix_MotorControl_RefNumRegistryGet.vi"("refnum name"="Turn3") -> ("error out"=w118:errorcluster, "PhoenixMotorControlDevRef"=w119:T10)  [unwired: 9 in]
          n93 = call-poly "CTRE_Phoenix_MotorController_Get_Enhanced.vi"("PhoenixMotorControlDevRef"=w119, "error in"=w118) -> ("Position (Raw Sensor Units)"=w114:i32)  [unwired: 10 in, 3 out]
          n94 = call-poly "CTRE_Phoenix_MotorController_Get_Enhanced.vi"("PhoenixMotorControlDevRef"=w121, "error in"=w120) -> ("Position (Raw Sensor Units)"=w115:i32)  [unwired: 10 in, 3 out]
          n95 = local write "Rel Pos 2"(w115) -> ()
          n96 = local write "Rel Pos 3"(w114) -> ()
        }
        frame #3 {
          w151 = T6 1 items=["PercentOutput"=0, "Position"=1, "Velocity"=2, "Current"=3, "Follower"=5, "MotionProfile"=6, "MotionMagic"=7, "MotionMagicArc"=8, "MotionProfileArc"=10, "Disabled"=15] ("Control Mode")
          w163 = T6 1 items=["PercentOutput"=0, "Position"=1, "Velocity"=2, "Current"=3, "Follower"=5, "MotionProfile"=6, "MotionMagic"=7, "MotionMagicArc"=8, "MotionProfileArc"=10, "Disabled"=15] ("Control Mode")
          # "Preps for Quad mode"
          n97 = local read "Current Pos 0"() -> (w131:dbl)
          n98 = local read "Start Pos 0"() -> (w149:i32)
          n99 = local read "Current Pos 1"() -> (w136:dbl)
          n100 = local read "Start Pos 1"() -> (w148:i32)
          n101 = local read "Current Pos 2"() -> (w138:dbl)
          n102 = local read "Current Pos 3"() -> (w139:dbl)
          n103 = local read "Start Pos 2"() -> (w147:i32)
          n104 = local read "Start Pos 3"() -> (w146:i32)
          n105 = call "CTRE_Phoenix_MotorControl_RefNumRegistryGet.vi"("refnum name"="Turn0") -> ("error out"=w171:errorcluster, "PhoenixMotorControlDevRef"=w170:T10)  [unwired: 9 in]
          n106 = call "CTRE_Phoenix_MotorControl_RefNumRegistryGet.vi"("refnum name"="Turn1") -> ("error out"=w169:errorcluster, "PhoenixMotorControlDevRef"=w168:T10)  [unwired: 9 in]
          n107 = call "CTRE_Phoenix_MotorControl_RefNumRegistryGet.vi"("refnum name"="Turn2") -> ("error out"=w167:errorcluster, "PhoenixMotorControlDevRef"=w166:T10)  [unwired: 9 in]
          n108 = call "CTRE_Phoenix_MotorControl_RefNumRegistryGet.vi"("refnum name"="Turn3") -> ("error out"=w165:errorcluster, "PhoenixMotorControlDevRef"=w164:T10)  [unwired: 9 in]
          n109 = Quotient & Remainder(x=w149, y=4096) -> (x-y*floor(x/y)=w132:i32)  [unwired: 1 out]
          n110 = Quotient & Remainder(x=w148, y=4096) -> (x-y*floor(x/y)=w137:i32)  [unwired: 1 out]
          n111 = Quotient & Remainder(x=w147, y=4096) -> (x-y*floor(x/y)=w141:i32)  [unwired: 1 out]
          n112 = Quotient & Remainder(x=w146, y=4096) -> (x-y*floor(x/y)=w140:i32)  [unwired: 1 out]
          n113 = Subtract(x=w136, y=w137) -> (x-y=w135:dbl)
          n114 = call "CTRE_Phoenix_MotorControl_SetSelectedSensorPosition.vi"("error in (no error)"=w169, "New Sensor Position"=w135, "PhoenixMotorControlDevRef"=w168) -> ("error out"=w159:errorcluster, "PhoenixMotorControlDevRef"=w160:T10)  [unwired: 7 in]
          n115 = Subtract(x=w131, y=w132) -> (x-y=w130:dbl)
          n116 = call "CTRE_Phoenix_MotorControl_SetSelectedSensorPosition.vi"("error in (no error)"=w171, "New Sensor Position"=w130, "PhoenixMotorControlDevRef"=w170) -> ("error out"=w161:errorcluster, "PhoenixMotorControlDevRef"=w162:T10)  [unwired: 7 in]
          n117 = Subtract(x=w138, y=w141) -> (x-y=w134:dbl)
          n118 = call "CTRE_Phoenix_MotorControl_SetSelectedSensorPosition.vi"("error in (no error)"=w167, "New Sensor Position"=w134, "PhoenixMotorControlDevRef"=w166) -> ("error out"=w157:errorcluster, "PhoenixMotorControlDevRef"=w158:T10)  [unwired: 7 in]
          n119 = Subtract(x=w139, y=w140) -> (x-y=w133:dbl)
          n120 = call "CTRE_Phoenix_MotorControl_SetSelectedSensorPosition.vi"("error in (no error)"=w165, "New Sensor Position"=w133, "PhoenixMotorControlDevRef"=w164) -> ("error out"=w155:errorcluster, "PhoenixMotorControlDevRef"=w156:T10)  [unwired: 7 in]
          n121 = call "CTRE_Phoenix_MotorControl_Set.vi"("error in (no error)"=w161, "Output"=w130, "Control Mode"=w163, "PhoenixMotorControlDevRef"=w162) -> ()  [unwired: 6 in, 2 out]
          n122 = call "CTRE_Phoenix_MotorControl_Set.vi"("error in (no error)"=w159, "Output"=w135, "Control Mode"=w163, "PhoenixMotorControlDevRef"=w160) -> ()  [unwired: 6 in, 2 out]
          n123 = call "CTRE_Phoenix_MotorControl_Set.vi"("error in (no error)"=w157, "Output"=w134, "Control Mode"=w163, "PhoenixMotorControlDevRef"=w158) -> ()  [unwired: 6 in, 2 out]
          n124 = call "CTRE_Phoenix_MotorControl_Set.vi"("error in (no error)"=w155, "Output"=w133, "Control Mode"=w163, "PhoenixMotorControlDevRef"=w156) -> ()  [unwired: 6 in, 2 out]
          n125 = call "CTRE_Phoenix_MotorControl_RefNumRegistryGet.vi"("refnum name"="IntakeUp") -> ("PhoenixMotorControlDevRef"=w154:T10)  [unwired: 9 in, 1 out]
          n126 = call "CTRE_Phoenix_MotorControl_Set.vi"("Output"=-4500.0, "Control Mode"=w151, "PhoenixMotorControlDevRef"=w154) -> ("PhoenixMotorControlDevRef"=w153:T10)  [unwired: 7 in, 1 out]
          n127 = call-poly "CTRE_Phoenix_MotorController_Get_Enhanced.vi"("PhoenixMotorControlDevRef"=w153) -> ()  [unwired: 9 in, 6 out]
        }
        frame #4 {
          n128 = call "CTRE_Phoenix_MotorControl_RefNumRegistryGet.vi"("refnum name"="Turn0") -> ("error out"=w186:errorcluster, "PhoenixMotorControlDevRef"=w187:T10)  [unwired: 9 in]
          n129 = call "CTRE_Phoenix_MotorControl_RefNumRegistryGet.vi"("refnum name"="Turn1") -> ("error out"=w184:errorcluster, "PhoenixMotorControlDevRef"=w185:T10)  [unwired: 9 in]
          n130 = call-poly "CTRE_Phoenix_MotorController_Get_Enhanced.vi"("PhoenixMotorControlDevRef"=w187, "error in"=w186) -> ("Position (Raw Sensor Units)"=w179:i32)  [unwired: 10 in, 3 out]
          n131 = call-poly "CTRE_Phoenix_MotorController_Get_Enhanced.vi"("PhoenixMotorControlDevRef"=w185, "error in"=w184) -> ("Position (Raw Sensor Units)"=w178:i32)  [unwired: 10 in, 3 out]
          n132 = local write "Final Rel Pos 0"(w179) -> ()
          n133 = local write "Final Rel Pos 1"(w178) -> ()
          n134 = call "CTRE_Phoenix_MotorControl_RefNumRegistryGet.vi"("refnum name"="Turn2") -> ("error out"=w182:errorcluster, "PhoenixMotorControlDevRef"=w183:T10)  [unwired: 9 in]
          n135 = call "CTRE_Phoenix_MotorControl_RefNumRegistryGet.vi"("refnum name"="Turn3") -> ("error out"=w180:errorcluster, "PhoenixMotorControlDevRef"=w181:T10)  [unwired: 9 in]
          n136 = call-poly "CTRE_Phoenix_MotorController_Get_Enhanced.vi"("PhoenixMotorControlDevRef"=w181, "error in"=w180) -> ("Position (Raw Sensor Units)"=w176:i32)  [unwired: 10 in, 3 out]
          n137 = call-poly "CTRE_Phoenix_MotorController_Get_Enhanced.vi"("PhoenixMotorControlDevRef"=w183, "error in"=w182) -> ("Position (Raw Sensor Units)"=w177:i32)  [unwired: 10 in, 3 out]
          n138 = local write "Final Rel Pos 2"(w177) -> ()
          n139 = local write "Final Rel Pos 3"(w176) -> ()
        }
      }
    }
    frame #1 {
      # "Dial#\n\n\n1\n2\n3\n4\n5"
      # "Guide for Auton Switch\n\n  10- NOTHING\n  06- LEFT (DNW)\n  02-MIDDLE\n  -2- RIGHT\n  -6-\n-10- Cross the Line"
      n140 = local read "Autonomous Select"() -> (w192:dbl)
      n141 = Multiply(x=w192, y=10.0) -> (x*y=w195:dbl)
      n142 = Round To Nearest(number=w195) -> (nearest integer value=w193:dbl)
      n143 = case shown="2" w193 {
        frame 1, Default {
        }
        frame 2 {
          n144 = stacked-sequence {
            frame #0 {
              n145 = Wait (ms)(milliseconds to wait=u32 750) -> ()  [unwired: 1 out]
            }
            frame #1 {
              n146 = while {
                stop <- w216 stop-if-true
                w198 = T6 7 items=["PercentOutput"=0, "Position"=1, "Velocity"=2, "Current"=3, "Follower"=5, "MotionProfile"=6, "MotionMagic"=7, "MotionMagicArc"=8, "MotionProfileArc"=10, "Disabled"=15] ("Control Mode")
                w203 = 0.4
                w220 = T6 1 items=["PercentOutput"=0, "Position"=1, "Velocity"=2, "Current"=3, "Follower"=5, "MotionProfile"=6, "MotionMagic"=7, "MotionMagicArc"=8, "MotionProfileArc"=10, "Disabled"=15] ("Control Mode")
                w227 = T6 1 items=["PercentOutput"=0, "Position"=1, "Velocity"=2, "Current"=3, "Follower"=5, "MotionProfile"=6, "MotionMagic"=7, "MotionMagicArc"=8, "MotionProfileArc"=10, "Disabled"=15] ("Control Mode")
                w230 = T6 1 items=["PercentOutput"=0, "Position"=1, "Velocity"=2, "Current"=3, "Follower"=5, "MotionProfile"=6, "MotionMagic"=7, "MotionMagicArc"=8, "MotionProfileArc"=10, "Disabled"=15] ("Control Mode")
                w244 = T6 1 items=["PercentOutput"=0, "Position"=1, "Velocity"=2, "Current"=3, "Follower"=5, "MotionProfile"=6, "MotionMagic"=7, "MotionMagicArc"=8, "MotionProfileArc"=10, "Disabled"=15] ("Control Mode")
                # "Turns and Moves the robot based on calculations"
                n147 = local read "MidSwitchPosition"() -> (w214:dbl)
                n148 = call <vilib>:"WPI_GyroRefNum Registry Get.vi"("refnum name"="Gyro") -> ("GyroDevRef"=w213:T7)  [unwired: 9 in, 1 out]
                n149 = call "CTRE_Phoenix_MotorControl_RefNumRegistryGet.vi"("refnum name"="Turn0") -> ("error out"=w219:errorcluster, "PhoenixMotorControlDevRef"=w222:T10)  [unwired: 9 in]
                n150 = call <vilib>:"WPI_GyroGetAngle.vi"("GyroDevRef"=w213) -> ("Angle"=w209:dbl)  [unwired: 6 in, 4 out]
                n151 = call "CTRE_Phoenix_MotorControl_RefNumRegistryGet.vi"("refnum name"="Turn1") -> ("error out"=w245:errorcluster, "PhoenixMotorControlDevRef"=w235:T10)  [unwired: 9 in]
                n152 = call-poly "CTRE_Phoenix_MotorController_Get_Enhanced.vi"("PhoenixMotorControlDevRef"=w222) -> ("PhoenixMotorControlDevRef"=w223:T10)  [unwired: 11 in, 3 out]
                n153 = global read "Robot Global Data.vi" "Gyro Centre"() -> (w210:dbl)
                n154 = call-poly "CTRE_Phoenix_MotorController_Get_Enhanced.vi"("PhoenixMotorControlDevRef"=w235) -> ("PhoenixMotorControlDevRef"=w234:T10)  [unwired: 11 in, 3 out]
                n155 = Subtract(x=w209, y=w210) -> (x-y=w211:dbl)
                n156 = Divide(x=w211, y=360.0) -> (x/y=w212:dbl)
                n157 = Multiply(x=w212, y=4096.0) -> (x*y=w205:dbl)
                n158 = Add(x=w214, y=w205) -> (x+y=w215:dbl)
                n159 = call "CTRE_Phoenix_MotorControl_Set.vi"("error in (no error)"=w219, "Output"=w215, "Control Mode"=w220, "PhoenixMotorControlDevRef"=w223) -> ()  [unwired: 6 in, 2 out]
                n160 = call "CTRE_Phoenix_MotorControl_Set.vi"("error in (no error)"=w245, "Output"=w215, "Control Mode"=w244, "PhoenixMotorControlDevRef"=w234) -> ()  [unwired: 6 in, 2 out]
                n161 = local read "ElevatorSwitch"() -> (w202:dbl)
                n162 = call "CTRE_Phoenix_MotorControl_RefNumRegistryGet.vi"("refnum name"="Turn3") -> ("error out"=w228:errorcluster, "PhoenixMotorControlDevRef"=w225:T10)  [unwired: 9 in]
                n163 = call "CTRE_Phoenix_MotorControl_RefNumRegistryGet.vi"("refnum name"="Turn2") -> ("error out"=w229:errorcluster, "PhoenixMotorControlDevRef"=w232:T10)  [unwired: 9 in]
                n164 = local read "ElevatePos"() -> (w199:dbl)
                n165 = call-poly "CTRE_Phoenix_MotorController_Get_Enhanced.vi"("PhoenixMotorControlDevRef"=w225) -> ("PhoenixMotorControlDevRef"=w224:T10)  [unwired: 11 in, 3 out]
                n166 = call-poly "CTRE_Phoenix_MotorController_Get_Enhanced.vi"("PhoenixMotorControlDevRef"=w232) -> ("PhoenixMotorControlDevRef"=w233:T10)  [unwired: 11 in, 3 out]
                n167 = call "CTRE_Phoenix_MotorControl_RefNumRegistryGet.vi"("refnum name"="Elevator") -> ("PhoenixMotorControlDevRef"=w200:T10)  [unwired: 9 in, 1 out]
                n168 = local write "ElevatePos"(w202) -> ()
                n169 = call "CTRE_Phoenix_MotorControl_Set.vi"("Output"=w199, "Control Mode"=w198, "PhoenixMotorControlDevRef"=w200) -> ()  [unwired: 7 in, 2 out]
                n170 = local read "MidSwitchPosition"() -> (w197:dbl)
                n171 = call "CTRE_Phoenix_MotorControl_Set.vi"("error in (no error)"=w228, "Output"=w215, "Control Mode"=w227, "PhoenixMotorControlDevRef"=w224) -> ()  [unwired: 6 in, 2 out]
                n172 = call "CTRE_Phoenix_MotorControl_Set.vi"("error in (no error)"=w229, "Output"=w215, "Control Mode"=w230, "PhoenixMotorControlDevRef"=w233) -> ()  [unwired: 6 in, 2 out]
                n173 = local write "Direction"(w197) -> ()
                n174 = call "Elapsed Time"("Time Target (s)"=1.5, "Set Start Time (s)"=0.0) -> ("Time has Elapsed"=w216:bool)  [unwired: 10 in, 7 out]
                n175 = call "CTRE_Phoenix_MotorControl_RefNumRegistryGet.vi"("refnum name"="Drive3") -> ("PhoenixMotorControlDevRef"=w240:T10)  [unwired: 9 in, 1 out]
                n176 = call "CTRE_Phoenix_MotorControl_RefNumRegistryGet.vi"("refnum name"="Drive2") -> ("PhoenixMotorControlDevRef"=w241:T10)  [unwired: 9 in, 1 out]
                n177 = call "CTRE_Phoenix_MotorControl_RefNumRegistryGet.vi"("refnum name"="Drive1") -> ("PhoenixMotorControlDevRef"=w242:T10)  [unwired: 9 in, 1 out]
                n178 = call "CTRE_Phoenix_MotorControl_RefNumRegistryGet.vi"("refnum name"="Drive0") -> ("PhoenixMotorControlDevRef"=w243:T10)  [unwired: 9 in, 1 out]
                n179 = local write "speed"(w203) -> ()
                n180 = call <vilib>:"WPI_MotorControlSetOutput.vi"("Output"=w203, "MotorControlDevRef"=w240) -> ()  [unwired: 7 in, 3 out]
                n181 = call <vilib>:"WPI_MotorControlSetOutput.vi"("Output"=w203, "MotorControlDevRef"=w241) -> ()  [unwired: 7 in, 3 out]
                n182 = call <vilib>:"WPI_MotorControlSetOutput.vi"("Output"=w203, "MotorControlDevRef"=w242) -> ()  [unwired: 7 in, 3 out]
                n183 = call <vilib>:"WPI_MotorControlSetOutput.vi"("Output"=w203, "MotorControlDevRef"=w243) -> ()  [unwired: 7 in, 3 out]
              }
            }
            frame #2 {
              w248 = u16 0 items=["None", "XON/XOFF", "RTS/CTS", "XON/XOFF & RTS/CTS", "DTR/DSR", "XON/XOFF & DTR/DSR"] ("Flow Control")
              w249 = u16 10 items=["1.0"=10, "1.5"=15, "2.0"=20] ("Stop Bits")
              w250 = u16 0 items=["None", "Odd", "Even", "Mark", "Space"] ("Parity")
              n184 = local write "speed"(0.4 ("speed")) -> ()
              n185 = call <vilib>:"WPI_SerialPortOpen.vi"("Baud Rate"=u32 9600, "Data Bits"=u16 8, "Parity"=w250, "Stop Bits"=w249, "Flow Control"=w248, "Serial Port"=WPI_SerialPort."Onboard RS-232") -> ("SerialPortRef"=w253:T19)  [unwired: 8 in, 1 out]
              n186 = call <vilib>:"WPI_SerialPortReset.vi"("SerialPortRef"=w253) -> ()  [unwired: 9 in, 2 out]
              n187 = while {
                stop <- FALSE stop-if-true
                w256 = T6 7 items=["PercentOutput"=0, "Position"=1, "Velocity"=2, "Current"=3, "Follower"=5, "MotionProfile"=6, "MotionMagic"=7, "MotionMagicArc"=8, "MotionProfileArc"=10, "Disabled"=15] ("Control Mode")
                w276 = T6 1 items=["PercentOutput"=0, "Position"=1, "Velocity"=2, "Current"=3, "Follower"=5, "MotionProfile"=6, "MotionMagic"=7, "MotionMagicArc"=8, "MotionProfileArc"=10, "Disabled"=15] ("Control Mode")
                w283 = T6 1 items=["PercentOutput"=0, "Position"=1, "Velocity"=2, "Current"=3, "Follower"=5, "MotionProfile"=6, "MotionMagic"=7, "MotionMagicArc"=8, "MotionProfileArc"=10, "Disabled"=15] ("Control Mode")
                w286 = T6 1 items=["PercentOutput"=0, "Position"=1, "Velocity"=2, "Current"=3, "Follower"=5, "MotionProfile"=6, "MotionMagic"=7, "MotionMagicArc"=8, "MotionProfileArc"=10, "Disabled"=15] ("Control Mode")
                w300 = T6 1 items=["PercentOutput"=0, "Position"=1, "Velocity"=2, "Current"=3, "Follower"=5, "MotionProfile"=6, "MotionMagic"=7, "MotionMagicArc"=8, "MotionProfileArc"=10, "Disabled"=15] ("Control Mode")
                # "Turns and Moves the robot based on calculations"
                n188 = call "CTRE_Phoenix_MotorControl_RefNumRegistryGet.vi"("refnum name"="Turn0") -> ("error out"=w275:errorcluster, "PhoenixMotorControlDevRef"=w278:T10)  [unwired: 9 in]
                n189 = call <vilib>:"WPI_GyroRefNum Registry Get.vi"("refnum name"="Gyro") -> ("GyroDevRef"=w268:T7)  [unwired: 9 in, 1 out]
                n190 = call "CTRE_Phoenix_MotorControl_RefNumRegistryGet.vi"("refnum name"="Turn1") -> ("error out"=w301:errorcluster, "PhoenixMotorControlDevRef"=w291:T10)  [unwired: 9 in]
                n191 = call-poly "CTRE_Phoenix_MotorController_Get_Enhanced.vi"("PhoenixMotorControlDevRef"=w278) -> ("PhoenixMotorControlDevRef"=w279:T10)  [unwired: 11 in, 3 out]
                n192 = call-poly "CTRE_Phoenix_MotorController_Get_Enhanced.vi"("PhoenixMotorControlDevRef"=w291) -> ("PhoenixMotorControlDevRef"=w290:T10)  [unwired: 11 in, 3 out]
                n193 = call <vilib>:"WPI_GyroGetAngle.vi"("GyroDevRef"=w268) -> ("Angle"=w267:dbl)  [unwired: 6 in, 4 out]
                n194 = global read "Robot Global Data.vi" "Gyro Centre"() -> (w271:dbl)
                n195 = local read "ElevatePos"() -> (w255:dbl)
                n196 = call "CTRE_Phoenix_MotorControl_RefNumRegistryGet.vi"("refnum name"="Elevator") -> ("PhoenixMotorControlDevRef"=w257:T10)  [unwired: 9 in, 1 out]
                n197 = Subtract(x=w267, y=w271) -> (x-y=w272:dbl)
                n198 = local read "Direction"() -> (w264:dbl)
                n199 = call "CTRE_Phoenix_MotorControl_Set.vi"("Output"=w255, "Control Mode"=w256, "PhoenixMotorControlDevRef"=w257) -> ()  [unwired: 7 in, 2 out]
                n200 = Divide(x=w272, y=360.0) -> (x/y=w273:dbl)
                n201 = Multiply(x=w273, y=4096.0) -> (x*y=w265:dbl)
                n202 = call "CTRE_Phoenix_MotorControl_RefNumRegistryGet.vi"("refnum name"="Turn3") -> ("error out"=w284:errorcluster, "PhoenixMotorControlDevRef"=w281:T10)  [unwired: 9 in]
                n203 = call "CTRE_Phoenix_MotorControl_RefNumRegistryGet.vi"("refnum name"="Turn2") -> ("error out"=w285:errorcluster, "PhoenixMotorControlDevRef"=w288:T10)  [unwired: 9 in]
                n204 = Add(x=w264, y=w265) -> (x+y=w263:dbl)
                n205 = call "CTRE_Phoenix_MotorControl_Set.vi"("error in (no error)"=w275, "Output"=w263, "Control Mode"=w276, "PhoenixMotorControlDevRef"=w279) -> ()  [unwired: 6 in, 2 out]
                n206 = call "CTRE_Phoenix_MotorControl_Set.vi"("error in (no error)"=w301, "Output"=w263, "Control Mode"=w300, "PhoenixMotorControlDevRef"=w290) -> ()  [unwired: 6 in, 2 out]
                n207 = call-poly "CTRE_Phoenix_MotorController_Get_Enhanced.vi"("PhoenixMotorControlDevRef"=w281) -> ("PhoenixMotorControlDevRef"=w280:T10)  [unwired: 11 in, 3 out]
                n208 = call-poly "CTRE_Phoenix_MotorController_Get_Enhanced.vi"("PhoenixMotorControlDevRef"=w288) -> ("PhoenixMotorControlDevRef"=w289:T10)  [unwired: 11 in, 3 out]
                n209 = call "CTRE_Phoenix_MotorControl_Set.vi"("error in (no error)"=w284, "Output"=w263, "Control Mode"=w283, "PhoenixMotorControlDevRef"=w280) -> ()  [unwired: 6 in, 2 out]
                n210 = call "CTRE_Phoenix_MotorControl_Set.vi"("error in (no error)"=w285, "Output"=w263, "Control Mode"=w286, "PhoenixMotorControlDevRef"=w289) -> ()  [unwired: 6 in, 2 out]
                n211 = call "Elapsed Time15"("Time Target (s)"=3.0, "Set Start Time (s)"=0.0) -> ("Time has Elapsed"=w261:bool)  [unwired: 10 in, 7 out]
                n212 = local read "speed"() -> (w274:dbl)
                n213 = call "CTRE_Phoenix_MotorControl_RefNumRegistryGet.vi"("refnum name"="Drive3") -> ("PhoenixMotorControlDevRef"=w296:T10)  [unwired: 9 in, 1 out]
                n214 = call "CTRE_Phoenix_MotorControl_RefNumRegistryGet.vi"("refnum name"="Drive2") -> ("PhoenixMotorControlDevRef"=w297:T10)  [unwired: 9 in, 1 out]
                n215 = call "CTRE_Phoenix_MotorControl_RefNumRegistryGet.vi"("refnum name"="Drive1") -> ("PhoenixMotorControlDevRef"=w298:T10)  [unwired: 9 in, 1 out]
                n216 = call "CTRE_Phoenix_MotorControl_RefNumRegistryGet.vi"("refnum name"="Drive0") -> ("PhoenixMotorControlDevRef"=w299:T10)  [unwired: 9 in, 1 out]
                n217 = case shown="True" w261 {
                  frame False {
                  }
                  frame True {
                    n218 = local write "speed"(0.0 ("speed")) -> ()
                    n219 = local write "stopped"(TRUE ("stopped")) -> ()
                  }
                }
                n220 = call <vilib>:"WPI_MotorControlSetOutput.vi"("Output"=w274, "MotorControlDevRef"=w296) -> ()  [unwired: 7 in, 3 out]
                n221 = call <vilib>:"WPI_MotorControlSetOutput.vi"("Output"=w274, "MotorControlDevRef"=w297) -> ()  [unwired: 7 in, 3 out]
                n222 = call <vilib>:"WPI_MotorControlSetOutput.vi"("Output"=w274, "MotorControlDevRef"=w298) -> ()  [unwired: 7 in, 3 out]
                n223 = call <vilib>:"WPI_MotorControlSetOutput.vi"("Output"=w274, "MotorControlDevRef"=w299) -> ()  [unwired: 7 in, 3 out]
              }
              n224 = while {
                shift-right: [w310] -> w254
                shift-left: w253 -> [w309]
                stop <- w306 stop-if-true
                # "Runs loop for about 116 days"
                # "Actual Auton"
                n225 = local read "stopped"() -> (w305:bool)
                n226 = case shown="True" w305 {
                  tunnel: [w312 w352] -> w310
                  tunnel: w309 -> [w311 w352]
                  frame False {
                    # "Auton 1: Basic Switch"
                    n227 = stacked-sequence {
                      tunnel: [w314 _ _] -> w312
                      tunnel: w311 -> [w313 _ _]
                      frame #0 {
                        n228 = while {
                          tunnel: [w325] -> w314
                          tunnel: w313 -> [w320]
                          stop <- w315 stop-if-true
                          # "Stops loop"
                          n229 = call <vilib>:"WPI_SerialPortGetBytesReceived.vi"("SerialPortRef"=w320) -> ("Bytes at Port"=w328:u32, "SerialPortRef"=w326:T19)  [unwired: 8 in, 1 out]
                          n230 = Greater Than 0?(x=w328) -> (x > 0?=w327:bool)
                          n231 = case shown="True" w327 {
                            tunnel: w328 -> [_ w335]
                            tunnel: w326 -> [w329 w334]
                            tunnel: [w329 w330] -> w325
                            frame False {
                            }
                            frame True {
                              # "Reads some stuff if we get some stuff"
                              n232 = local read "Text"() -> (w332:string)
                              n233 = call <vilib>:"WPI_SerialPortRead.vi"("Num Bytes to Read"=w335, "SerialPortRef"=w334) -> ("Buffer"=w331:string, "SerialPortRef"=w330:T19)  [unwired: 7 in, 1 out]
                              n234 = Concatenate Strings(w332, w331) -> (w333:string)
                              n235 = local write "Text"(w333) -> ()
                              n236 = local write "Current Reading"(w331) -> ()
                            }
                          }
                          n237 = local read "Text"() -> (w324:string)
                          n238 = Match Pattern(string=w324, regular expression="\\n") -> (offset past match=w322:i32)  [unwired: 1 in, 3 out]
                          n239 = Greater?(x=w322, y=-1) -> (0:w316:bool)
                          n240 = call "Elapsed Time2"("Time Target (s)"=3.0, "Set Start Time (s)"=0.0) -> ("Time has Elapsed"=w317:bool)  [unwired: 10 in, 7 out]
                          n241 = Or(x=w317, y=w316) -> (x .or. y?=w315:bool)
                        }
                      }
                      frame #1 {
                        # "Gives X (Left and Right) and Z (Distance)"
                        n242 = local read "Text"() -> (w341:string)
                        n243 = Match Pattern(string=w341, regular expression=",") -> (after substring=w339:string)  [unwired: 1 in, 3 out]
                        n244 = Match Pattern(string=w339, regular expression=",") -> (before substring=w337:string)  [unwired: 1 in, 3 out]
                        n245 = Decimal String To Number(string=w337) -> (number=w336:i32)  [unwired: 2 in, 1 out]
                        n246 = local write "x"(w336) -> ()
                      }
                      frame #2 {
                        # "Gives Direction to go!"
                        n247 = local read "x"() -> (w343:dbl)
                        n248 = Greater Than 0?(x=w343) -> (x > 0?=w342:bool)
                        n249 = local write "Text"("") -> ()
                        n250 = case shown="True" w342 {
                          frame False {
                          }
                          frame True {
                            n251 = local read "x"() -> (w349:dbl)
                            n252 = Divide(x=w349, y=320.0) -> (x/y=w348:dbl)
                            n253 = Multiply(x=w348, y=1800.0) -> (x*y=w350:dbl)
                            n254 = Subtract(x=900.0, y=w350) -> (x-y=w351:dbl)
                            n255 = local write "Direction"(w351) -> ()
                          }
                        }
                      }
                    }
                  }
                  frame True {
                    n256 = local read "CoolDown"() -> (w353:bool)
                    n257 = case shown="False" w353 {
                      tunnel: w352 -> [w354 _]
                      frame False {
                        n258 = stacked-sequence {
                          tunnel: w354 -> [_ _ _ _ _ _ w426 _ _ _]
                          frame #0 {
                            w355 = 1.0
                            n259 = local write "Direction"(0.0 ("Direction")) -> ()
                            n260 = local write "speed"(0.0 ("speed")) -> ()
                            n261 = call "CTRE_Phoenix_MotorControl_RefNumRegistryGet.vi"("refnum name"="Intake1") -> ("PhoenixMotorControlDevRef"=w356:T10)  [unwired: 9 in, 1 out]
                            n262 = call "CTRE_Phoenix_MotorControl_RefNumRegistryGet.vi"("refnum name"="Intake2") -> ("PhoenixMotorControlDevRef"=w359:T10)  [unwired: 9 in, 1 out]
                            n263 = Negate(x=w355) -> (-x=w360:dbl)
                            n264 = call <vilib>:"WPI_MotorControlSetOutput.vi"("Output"=w355, "MotorControlDevRef"=w359) -> ()  [unwired: 7 in, 3 out]
                            n265 = call <vilib>:"WPI_MotorControlSetOutput.vi"("Output"=w360, "MotorControlDevRef"=w356) -> ()  [unwired: 7 in, 3 out]
                            n266 = Wait (ms)(milliseconds to wait=u32 500) -> ()  [unwired: 1 out]
                          }
                          frame #1 {
                            n267 = while {
                              stop <- w370 stop-if-true
                              w364 = 0.0
                              n268 = call "CTRE_Phoenix_MotorControl_RefNumRegistryGet.vi"("refnum name"="Intake1") -> ("PhoenixMotorControlDevRef"=w365:T10)  [unwired: 9 in, 1 out]
                              n269 = call "CTRE_Phoenix_MotorControl_RefNumRegistryGet.vi"("refnum name"="Intake2") -> ("PhoenixMotorControlDevRef"=w368:T10)  [unwired: 9 in, 1 out]
                              n270 = local write "Direction"(2048.0 ("Direction")) -> ()
                              n271 = local write "speed"(0.5 ("speed")) -> ()
                              n272 = Negate(x=w364) -> (-x=w369:dbl)
                              n273 = call <vilib>:"WPI_MotorControlSetOutput.vi"("Output"=w364, "MotorControlDevRef"=w368) -> ()  [unwired: 7 in, 3 out]
                              n274 = call <vilib>:"WPI_MotorControlSetOutput.vi"("Output"=w369, "MotorControlDevRef"=w365) -> ()  [unwired: 7 in, 3 out]
                              n275 = call "Elapsed Time14"("Time Target (s)"=1.5, "Set Start Time (s)"=0.0) -> ("Time has Elapsed"=w370:bool)  [unwired: 10 in, 7 out]
                            }
                          }
                          frame #2 {
                            n276 = while {
                              stop <- w380 stop-if-true
                              n277 = local read "Switch"() -> (w377:bool)
                              n278 = Select(t=3072.0 ("Direction"), s=w377, f=1024.0) -> (s? t:f=w375:dbl)
                              n279 = local write "speed"(0.6 ("speed")) -> ()
                              n280 = local write "Direction"(w375) -> ()
                              n281 = local read "ElevatorDown"() -> (w379:dbl)
                              n282 = local write "ElevatePos"(w379) -> ()
                              n283 = call "Elapsed Time19"("Time Target (s)"=1.15, "Set Start Time (s)"=0.0) -> ("Time has Elapsed"=w380:bool)  [unwired: 10 in, 7 out]
                            }
                          }
                          frame #3 {
                            n284 = while {
                              stop <- w394 stop-if-true
                              w389 = -1.0
                              n285 = local write "speed"(0.4 ("speed")) -> ()
                              n286 = local write "Direction"(0.0 ("Direction")) -> ()
                              n287 = call "CTRE_Phoenix_MotorControl_RefNumRegistryGet.vi"("refnum name"="Intake1") -> ("PhoenixMotorControlDevRef"=w392:T10)  [unwired: 9 in, 1 out]
                              n288 = call "CTRE_Phoenix_MotorControl_RefNumRegistryGet.vi"("refnum name"="Intake2") -> ("PhoenixMotorControlDevRef"=w391:T10)  [unwired: 9 in, 1 out]
                              n289 = Negate(x=w389) -> (-x=w390:dbl)
                              n290 = call <vilib>:"WPI_MotorControlSetOutput.vi"("Output"=w389, "MotorControlDevRef"=w391) -> ()  [unwired: 7 in, 3 out]
                              n291 = call <vilib>:"WPI_MotorControlSetOutput.vi"("Output"=w390, "MotorControlDevRef"=w392) -> ()  [unwired: 7 in, 3 out]
                              n292 = call "Elapsed Time6"("Time Target (s)"=0.75, "Set Start Time (s)"=0.0) -> ("Time has Elapsed"=w394:bool)  [unwired: 10 in, 7 out]
                              n293 = call <vilib>:"WPI_SolenoidRefNum Registry Get.vi"("refnum name"="Open/Close") -> ("SolenoidDevRef"=w386:T20)  [unwired: 9 in, 1 out]
                              n294 = call-poly <vilib>:"WPI_SolenoidSet.vi"("Value"=TRUE, "SolenoidDevRef"=w386) -> ()  [unwired: 8 in, 2 out]
                            }
                          }
                          frame #4 {
                            n295 = while {
                              stop <- w411 stop-if-true
                              w407 = -1.0
                              n296 = local read "Switch"() -> (w399:bool)
                              n297 = Select(t=1024.0 ("Direction"), s=w399, f=3072.0) -> (s? t:f=w400:dbl)
                              n298 = local write "speed"(0.0 ("speed")) -> ()
                              n299 = local write "Direction"(w400) -> ()
                              n300 = call "CTRE_Phoenix_MotorControl_RefNumRegistryGet.vi"("refnum name"="Intake1") -> ("PhoenixMotorControlDevRef"=w410:T10)  [unwired: 9 in, 1 out]
                              n301 = call "CTRE_Phoenix_MotorControl_RefNumRegistryGet.vi"("refnum name"="Intake2") -> ("PhoenixMotorControlDevRef"=w409:T10)  [unwired: 9 in, 1 out]
                              n302 = Negate(x=w407) -> (-x=w408:dbl)
                              n303 = call <vilib>:"WPI_MotorControlSetOutput.vi"("Output"=w407, "MotorControlDevRef"=w409) -> ()  [unwired: 7 in, 3 out]
                              n304 = call <vilib>:"WPI_MotorControlSetOutput.vi"("Output"=w408, "MotorControlDevRef"=w410) -> ()  [unwired: 7 in, 3 out]
                              n305 = call "Elapsed Time20"("Time Target (s)"=0.5, "Set Start Time (s)"=0.0) -> ("Time has Elapsed"=w411:bool)  [unwired: 10 in, 7 out]
                              n306 = call <vilib>:"WPI_SolenoidRefNum Registry Get.vi"("refnum name"="Open/Close") -> ("SolenoidDevRef"=w404:T20)  [unwired: 9 in, 1 out]
                              n307 = call-poly <vilib>:"WPI_SolenoidSet.vi"("Value"=FALSE, "SolenoidDevRef"=w404) -> ()  [unwired: 8 in, 2 out]
                            }
                          }
                          frame #5 {
                            n308 = while {
                              stop <- w422 stop-if-true
                              w418 = 0.0
                              n309 = local read "ElevatorSwitch"() -> (w415:dbl)
                              n310 = local write "speed"(0.5 ("speed")) -> ()
                              n311 = local write "ElevatePos"(w415) -> ()
                              n312 = call "CTRE_Phoenix_MotorControl_RefNumRegistryGet.vi"("refnum name"="Intake1") -> ("PhoenixMotorControlDevRef"=w421:T10)  [unwired: 9 in, 1 out]
                              n313 = call "CTRE_Phoenix_MotorControl_RefNumRegistryGet.vi"("refnum name"="Intake2") -> ("PhoenixMotorControlDevRef"=w420:T10)  [unwired: 9 in, 1 out]
                              n314 = Negate(x=w418) -> (-x=w419:dbl)
                              n315 = call <vilib>:"WPI_MotorControlSetOutput.vi"("Output"=w418, "MotorControlDevRef"=w420) -> ()  [unwired: 7 in, 3 out]
                              n316 = call <vilib>:"WPI_MotorControlSetOutput.vi"("Output"=w419, "MotorControlDevRef"=w421) -> ()  [unwired: 7 in, 3 out]
                              n317 = call "Elapsed Time26"("Time Target (s)"=1.5, "Set Start Time (s)"=0.0) -> ("Time has Elapsed"=w422:bool)  [unwired: 10 in, 7 out]
                            }
                          }
                          frame #6 {
                            n318 = while {
                              tunnel: w426 -> [w427]
                              stop <- w428 stop-if-true
                              n319 = stacked-sequence {
                                tunnel: [w433 _ _] -> _
                                tunnel: w427 -> [w432 _ _]
                                frame #0 {
                                n320 = while {
                                tunnel: [w444] -> w433
                                tunnel: w432 -> [w434]
                                stop <- w435 stop-if-true
                                # "Stops loop"
                                n321 = call <vilib>:"WPI_SerialPortGetBytesReceived.vi"("SerialPortRef"=w434) -> ("Bytes at Port"=w447:u32, "SerialPortRef"=w445:T19)  [unwired: 8 in, 1 out]
                                n322 = Greater Than 0?(x=w447) -> (x > 0?=w446:bool)
                                n323 = case shown="True" w446 {
                                tunnel: w447 -> [_ w454]
                                tunnel: w445 -> [w448 w453]
                                tunnel: [w448 w449] -> w444
                                frame False {
                                }
                                frame True {
                                # "Reads some stuff if we get some stuff"
                                n324 = local read "Text"() -> (w451:string)
                                n325 = call <vilib>:"WPI_SerialPortRead.vi"("Num Bytes to Read"=w454, "SerialPortRef"=w453) -> ("Buffer"=w450:string, "SerialPortRef"=w449:T19)  [unwired: 7 in, 1 out]
                                n326 = Concatenate Strings(w451, w450) -> (w452:string)
                                n327 = local write "Text"(w452) -> ()
                                n328 = local write "Current Reading"(w450) -> ()
                                }
                                }
                                n329 = local read "Text"() -> (w443:string)
                                n330 = Match Pattern(string=w443, regular expression="\\n") -> (offset past match=w441:i32)  [unwired: 1 in, 3 out]
                                n331 = Greater?(x=w441, y=-1) -> (0:w436:bool)
                                n332 = call "Elapsed Time25"("Time Target (s)"=3.0, "Set Start Time (s)"=0.0) -> ("Time has Elapsed"=w437:bool)  [unwired: 10 in, 7 out]
                                n333 = Or(x=w437, y=w436) -> (x .or. y?=w435:bool)
                                }
                                }
                                frame #1 {
                                n334 = local read "Text"() -> (w460:string)
                                n335 = Match Pattern(string=w460, regular expression=",") -> (after substring=w458:string)  [unwired: 1 in, 3 out]
                                n336 = Match Pattern(string=w458, regular expression=",") -> (before substring=w456:string)  [unwired: 1 in, 3 out]
                                n337 = Decimal String To Number(string=w456) -> (number=w455:i32)  [unwired: 2 in, 1 out]
                                n338 = local write "x"(w455) -> ()
                                }
                                frame #2 {
                                # "Gives Direction to go!"
                                n339 = local read "x"() -> (w462:dbl)
                                n340 = Greater Than 0?(x=w462) -> (x > 0?=w461:bool)
                                n341 = local write "Text"("") -> ()
                                n342 = case shown="False" w461 {
                                frame False {
                                }
                                frame True {
                                n343 = local read "x"() -> (w468:dbl)
                                n344 = Divide(x=w468, y=320.0) -> (x/y=w467:dbl)
                                n345 = Multiply(x=w467, y=1800.0) -> (x*y=w469:dbl)
                                n346 = Subtract(x=900.0, y=w469) -> (x-y=w470:dbl)
                                n347 = local write "Direction"(w470) -> ()
                                }
                                }
                                }
                              }
                              n348 = local write "speed"(0.5 ("speed")) -> ()
                              n349 = call "Elapsed Time21"("Time Target (s)"=3.0, "Set Start Time (s)"=0.0) -> ("Time has Elapsed"=w428:bool)  [unwired: 10 in, 7 out]
                            }
                          }
                          frame #7 {
                            n350 = while {
                              stop <- w478 stop-if-true
                              w473 = 1.0
                              n351 = local write "speed"(0.0 ("speed")) -> ()
                              n352 = local write "Direction"(0.0 ("Direction")) -> ()
                              n353 = call "CTRE_Phoenix_MotorControl_RefNumRegistryGet.vi"("refnum name"="Intake1") -> ("PhoenixMotorControlDevRef"=w476:T10)  [unwired: 9 in, 1 out]
                              n354 = call "CTRE_Phoenix_MotorControl_RefNumRegistryGet.vi"("refnum name"="Intake2") -> ("PhoenixMotorControlDevRef"=w475:T10)  [unwired: 9 in, 1 out]
                              n355 = Negate(x=w473) -> (-x=w474:dbl)
                              n356 = call <vilib>:"WPI_MotorControlSetOutput.vi"("Output"=w473, "MotorControlDevRef"=w475) -> ()  [unwired: 7 in, 3 out]
                              n357 = call <vilib>:"WPI_MotorControlSetOutput.vi"("Output"=w474, "MotorControlDevRef"=w476) -> ()  [unwired: 7 in, 3 out]
                              n358 = call "Elapsed Time23"("Time Target (s)"=0.5, "Set Start Time (s)"=0.0) -> ("Time has Elapsed"=w478:bool)  [unwired: 10 in, 7 out]
                            }
                          }
                          frame #8 {
                            n359 = while {
                              stop <- w489 stop-if-true
                              w484 = 0.0
                              n360 = local write "speed"(0.6 ("speed")) -> ()
                              n361 = local write "Direction"(2048.0 ("Direction")) -> ()
                              n362 = call "CTRE_Phoenix_MotorControl_RefNumRegistryGet.vi"("refnum name"="Intake1") -> ("PhoenixMotorControlDevRef"=w487:T10)  [unwired: 9 in, 1 out]
                              n363 = call "CTRE_Phoenix_MotorControl_RefNumRegistryGet.vi"("refnum name"="Intake2") -> ("PhoenixMotorControlDevRef"=w486:T10)  [unwired: 9 in, 1 out]
                              n364 = Negate(x=w484) -> (-x=w485:dbl)
                              n365 = call <vilib>:"WPI_MotorControlSetOutput.vi"("Output"=w484, "MotorControlDevRef"=w486) -> ()  [unwired: 7 in, 3 out]
                              n366 = call <vilib>:"WPI_MotorControlSetOutput.vi"("Output"=w485, "MotorControlDevRef"=w487) -> ()  [unwired: 7 in, 3 out]
                              n367 = call "Elapsed Time24"("Time Target (s)"=1.5, "Set Start Time (s)"=0.0) -> ("Time has Elapsed"=w489:bool)  [unwired: 10 in, 7 out]
                            }
                          }
                          frame #9 {
                            n368 = local write "speed"(0.0 ("speed")) -> ()
                            n369 = local write "Direction"(0.0 ("Direction")) -> ()
                            n370 = local write "CoolDown"(TRUE ("CoolDown")) -> ()
                          }
                        }
                      }
                      frame True {
                      }
                    }
                  }
                }
                n371 = call "Elapsed Time3"("Time Target (s)"=14.5, "Set Start Time (s)"=0.0) -> ("Time has Elapsed"=w306:bool)  [unwired: 10 in, 7 out]
              }
              n372 = call <vilib>:"WPI_SerialPortClose.vi"("SerialPortRef"=w254) -> ()  [unwired: 10 in, 1 out]
            }
          }
        }
        frame -6 {
          # "Exchange"
          n373 = stacked-sequence {
            frame #0 {
              n374 = while {
                stop <- w515 stop-if-true
                w498 = T6 7 items=["PercentOutput"=0, "Position"=1, "Velocity"=2, "Current"=3, "Follower"=5, "MotionProfile"=6, "MotionMagic"=7, "MotionMagicArc"=8, "MotionProfileArc"=10, "Disabled"=15] ("Control Mode")
                w503 = 0.4
                w519 = T6 1 items=["PercentOutput"=0, "Position"=1, "Velocity"=2, "Current"=3, "Follower"=5, "MotionProfile"=6, "MotionMagic"=7, "MotionMagicArc"=8, "MotionProfileArc"=10, "Disabled"=15] ("Control Mode")
                w526 = T6 1 items=["PercentOutput"=0, "Position"=1, "Velocity"=2, "Current"=3, "Follower"=5, "MotionProfile"=6, "MotionMagic"=7, "MotionMagicArc"=8, "MotionProfileArc"=10, "Disabled"=15] ("Control Mode")
                w529 = T6 1 items=["PercentOutput"=0, "Position"=1, "Velocity"=2, "Current"=3, "Follower"=5, "MotionProfile"=6, "MotionMagic"=7, "MotionMagicArc"=8, "MotionProfileArc"=10, "Disabled"=15] ("Control Mode")
                w543 = T6 1 items=["PercentOutput"=0, "Position"=1, "Velocity"=2, "Current"=3, "Follower"=5, "MotionProfile"=6, "MotionMagic"=7, "MotionMagicArc"=8, "MotionProfileArc"=10, "Disabled"=15] ("Control Mode")
                # "Turns and Moves the robot based on calculations"
                n375 = call <vilib>:"WPI_GyroRefNum Registry Get.vi"("refnum name"="Gyro") -> ("GyroDevRef"=w513:T7)  [unwired: 9 in, 1 out]
                n376 = call "CTRE_Phoenix_MotorControl_RefNumRegistryGet.vi"("refnum name"="Turn0") -> ("error out"=w518:errorcluster, "PhoenixMotorControlDevRef"=w521:T10)  [unwired: 9 in]
                n377 = call <vilib>:"WPI_GyroGetAngle.vi"("GyroDevRef"=w513) -> ("Angle"=w509:dbl)  [unwired: 6 in, 4 out]
                n378 = call "CTRE_Phoenix_MotorControl_RefNumRegistryGet.vi"("refnum name"="Turn1") -> ("error out"=w544:errorcluster, "PhoenixMotorControlDevRef"=w534:T10)  [unwired: 9 in]
                n379 = call-poly "CTRE_Phoenix_MotorController_Get_Enhanced.vi"("PhoenixMotorControlDevRef"=w521) -> ("PhoenixMotorControlDevRef"=w522:T10)  [unwired: 11 in, 3 out]
                n380 = global read "Robot Global Data.vi" "Gyro Centre"() -> (w510:dbl)
                n381 = call-poly "CTRE_Phoenix_MotorController_Get_Enhanced.vi"("PhoenixMotorControlDevRef"=w534) -> ("PhoenixMotorControlDevRef"=w533:T10)  [unwired: 11 in, 3 out]
                n382 = Subtract(x=w509, y=w510) -> (x-y=w511:dbl)
                n383 = Divide(x=w511, y=360.0) -> (x/y=w512:dbl)
                n384 = Multiply(x=w512, y=4096.0) -> (x*y=w505:dbl)
                n385 = Add(x=-750.0, y=w505) -> (x+y=w514:dbl)
                n386 = call "CTRE_Phoenix_MotorControl_Set.vi"("error in (no error)"=w518, "Output"=w514, "Control Mode"=w519, "PhoenixMotorControlDevRef"=w522) -> ()  [unwired: 6 in, 2 out]
                n387 = call "CTRE_Phoenix_MotorControl_Set.vi"("error in (no error)"=w544, "Output"=w514, "Control Mode"=w543, "PhoenixMotorControlDevRef"=w533) -> ()  [unwired: 6 in, 2 out]
                n388 = local read "ElevatorSwitch"() -> (w502:dbl)
                n389 = call "CTRE_Phoenix_MotorControl_RefNumRegistryGet.vi"("refnum name"="Turn3") -> ("error out"=w527:errorcluster, "PhoenixMotorControlDevRef"=w524:T10)  [unwired: 9 in]
                n390 = call "CTRE_Phoenix_MotorControl_RefNumRegistryGet.vi"("refnum name"="Turn2") -> ("error out"=w528:errorcluster, "PhoenixMotorControlDevRef"=w531:T10)  [unwired: 9 in]
                n391 = local read "ElevatePos"() -> (w499:dbl)
                n392 = local read "MidSwitchPosition"() -> (w497:dbl)
                n393 = call-poly "CTRE_Phoenix_MotorController_Get_Enhanced.vi"("PhoenixMotorControlDevRef"=w524) -> ("PhoenixMotorControlDevRef"=w523:T10)  [unwired: 11 in, 3 out]
                n394 = call-poly "CTRE_Phoenix_MotorController_Get_Enhanced.vi"("PhoenixMotorControlDevRef"=w531) -> ("PhoenixMotorControlDevRef"=w532:T10)  [unwired: 11 in, 3 out]
                n395 = call "CTRE_Phoenix_MotorControl_RefNumRegistryGet.vi"("refnum name"="Elevator") -> ("PhoenixMotorControlDevRef"=w500:T10)  [unwired: 9 in, 1 out]
                n396 = local write "ElevatePos"(w502) -> ()
                n397 = call "CTRE_Phoenix_MotorControl_Set.vi"("Output"=w499, "Control Mode"=w498, "PhoenixMotorControlDevRef"=w500) -> ()  [unwired: 7 in, 2 out]
                n398 = local write "Direction"(w497) -> ()
                n399 = call "CTRE_Phoenix_MotorControl_Set.vi"("error in (no error)"=w527, "Output"=w514, "Control Mode"=w526, "PhoenixMotorControlDevRef"=w523) -> ()  [unwired: 6 in, 2 out]
                n400 = call "CTRE_Phoenix_MotorControl_Set.vi"("error in (no error)"=w528, "Output"=w514, "Control Mode"=w529, "PhoenixMotorControlDevRef"=w532) -> ()  [unwired: 6 in, 2 out]
                n401 = call "Elapsed Time7"("Time Target (s)"=1.5, "Set Start Time (s)"=0.0) -> ("Time has Elapsed"=w515:bool)  [unwired: 10 in, 7 out]
                n402 = call "CTRE_Phoenix_MotorControl_RefNumRegistryGet.vi"("refnum name"="Drive3") -> ("PhoenixMotorControlDevRef"=w539:T10)  [unwired: 9 in, 1 out]
                n403 = call "CTRE_Phoenix_MotorControl_RefNumRegistryGet.vi"("refnum name"="Drive2") -> ("PhoenixMotorControlDevRef"=w540:T10)  [unwired: 9 in, 1 out]
                n404 = call "CTRE_Phoenix_MotorControl_RefNumRegistryGet.vi"("refnum name"="Drive1") -> ("PhoenixMotorControlDevRef"=w541:T10)  [unwired: 9 in, 1 out]
                n405 = call "CTRE_Phoenix_MotorControl_RefNumRegistryGet.vi"("refnum name"="Drive0") -> ("PhoenixMotorControlDevRef"=w542:T10)  [unwired: 9 in, 1 out]
                n406 = local write "speed"(w503) -> ()
                n407 = call <vilib>:"WPI_MotorControlSetOutput.vi"("Output"=w503, "MotorControlDevRef"=w539) -> ()  [unwired: 7 in, 3 out]
                n408 = call <vilib>:"WPI_MotorControlSetOutput.vi"("Output"=w503, "MotorControlDevRef"=w540) -> ()  [unwired: 7 in, 3 out]
                n409 = call <vilib>:"WPI_MotorControlSetOutput.vi"("Output"=w503, "MotorControlDevRef"=w541) -> ()  [unwired: 7 in, 3 out]
                n410 = call <vilib>:"WPI_MotorControlSetOutput.vi"("Output"=w503, "MotorControlDevRef"=w542) -> ()  [unwired: 7 in, 3 out]
              }
            }
            frame #1 {
              w546 = u16 0 items=["None", "XON/XOFF", "RTS/CTS", "XON/XOFF & RTS/CTS", "DTR/DSR", "XON/XOFF & DTR/DSR"] ("Flow Control")
              w547 = u16 10 items=["1.0"=10, "1.5"=15, "2.0"=20] ("Stop Bits")
              w548 = u16 0 items=["None", "Odd", "Even", "Mark", "Space"] ("Parity")
              n411 = call <vilib>:"WPI_SerialPortOpen.vi"("Baud Rate"=u32 9600, "Data Bits"=u16 8, "Parity"=w548, "Stop Bits"=w547, "Flow Control"=w546, "Serial Port"=WPI_SerialPort."Onboard RS-232") -> ("SerialPortRef"=w551:T19)  [unwired: 8 in, 1 out]
              n412 = call <vilib>:"WPI_SerialPortReset.vi"("SerialPortRef"=w551) -> ()  [unwired: 9 in, 2 out]
              n413 = while {
                stop <- FALSE stop-if-true
                w555 = T6 7 items=["PercentOutput"=0, "Position"=1, "Velocity"=2, "Current"=3, "Follower"=5, "MotionProfile"=6, "MotionMagic"=7, "MotionMagicArc"=8, "MotionProfileArc"=10, "Disabled"=15] ("Control Mode")
                w574 = T6 1 items=["PercentOutput"=0, "Position"=1, "Velocity"=2, "Current"=3, "Follower"=5, "MotionProfile"=6, "MotionMagic"=7, "MotionMagicArc"=8, "MotionProfileArc"=10, "Disabled"=15] ("Control Mode")
                w581 = T6 1 items=["PercentOutput"=0, "Position"=1, "Velocity"=2, "Current"=3, "Follower"=5, "MotionProfile"=6, "MotionMagic"=7, "MotionMagicArc"=8, "MotionProfileArc"=10, "Disabled"=15] ("Control Mode")
                w584 = T6 1 items=["PercentOutput"=0, "Position"=1, "Velocity"=2, "Current"=3, "Follower"=5, "MotionProfile"=6, "MotionMagic"=7, "MotionMagicArc"=8, "MotionProfileArc"=10, "Disabled"=15] ("Control Mode")
                w598 = T6 1 items=["PercentOutput"=0, "Position"=1, "Velocity"=2, "Current"=3, "Follower"=5, "MotionProfile"=6, "MotionMagic"=7, "MotionMagicArc"=8, "MotionProfileArc"=10, "Disabled"=15] ("Control Mode")
                # "Where does this even come from?"
                # "Turns and Moves the robot based on calculations"
                n414 = call "CTRE_Phoenix_MotorControl_RefNumRegistryGet.vi"("refnum name"="Turn0") -> ("error out"=w573:errorcluster, "PhoenixMotorControlDevRef"=w576:T10)  [unwired: 9 in]
                n415 = call <vilib>:"WPI_GyroRefNum Registry Get.vi"("refnum name"="Gyro") -> ("GyroDevRef"=w566:T7)  [unwired: 9 in, 1 out]
                n416 = call "CTRE_Phoenix_MotorControl_RefNumRegistryGet.vi"("refnum name"="Turn1") -> ("error out"=w599:errorcluster, "PhoenixMotorControlDevRef"=w589:T10)  [unwired: 9 in]
                n417 = call-poly "CTRE_Phoenix_MotorController_Get_Enhanced.vi"("PhoenixMotorControlDevRef"=w576) -> ("PhoenixMotorControlDevRef"=w577:T10)  [unwired: 11 in, 3 out]
                n418 = call-poly "CTRE_Phoenix_MotorController_Get_Enhanced.vi"("PhoenixMotorControlDevRef"=w589) -> ("PhoenixMotorControlDevRef"=w588:T10)  [unwired: 11 in, 3 out]
                n419 = call <vilib>:"WPI_GyroGetAngle.vi"("GyroDevRef"=w566) -> ("Angle"=w565:dbl)  [unwired: 6 in, 4 out]
                n420 = global read "Robot Global Data.vi" "Gyro Centre"() -> (w569:dbl)
                n421 = local read "ElevatePos"() -> (w554:dbl)
                n422 = call "CTRE_Phoenix_MotorControl_RefNumRegistryGet.vi"("refnum name"="Elevator") -> ("PhoenixMotorControlDevRef"=w556:T10)  [unwired: 9 in, 1 out]
                n423 = Subtract(x=w565, y=w569) -> (x-y=w570:dbl)
                n424 = call "CTRE_Phoenix_MotorControl_Set.vi"("Output"=w554, "Control Mode"=w555, "PhoenixMotorControlDevRef"=w556) -> ()  [unwired: 7 in, 2 out]
                n425 = Divide(x=w570, y=360.0) -> (x/y=w571:dbl)
                n426 = Multiply(x=w571, y=4096.0) -> (x*y=w563:dbl)
                n427 = call "CTRE_Phoenix_MotorControl_RefNumRegistryGet.vi"("refnum name"="Turn3") -> ("error out"=w582:errorcluster, "PhoenixMotorControlDevRef"=w579:T10)  [unwired: 9 in]
                n428 = call "CTRE_Phoenix_MotorControl_RefNumRegistryGet.vi"("refnum name"="Turn2") -> ("error out"=w583:errorcluster, "PhoenixMotorControlDevRef"=w586:T10)  [unwired: 9 in]
                n429 = Add(x=1000.0, y=w563) -> (x+y=w562:dbl)
                n430 = call "CTRE_Phoenix_MotorControl_Set.vi"("error in (no error)"=w573, "Output"=w562, "Control Mode"=w574, "PhoenixMotorControlDevRef"=w577) -> ()  [unwired: 6 in, 2 out]
                n431 = call "CTRE_Phoenix_MotorControl_Set.vi"("error in (no error)"=w599, "Output"=w562, "Control Mode"=w598, "PhoenixMotorControlDevRef"=w588) -> ()  [unwired: 6 in, 2 out]
                n432 = call-poly "CTRE_Phoenix_MotorController_Get_Enhanced.vi"("PhoenixMotorControlDevRef"=w579) -> ("PhoenixMotorControlDevRef"=w578:T10)  [unwired: 11 in, 3 out]
                n433 = call-poly "CTRE_Phoenix_MotorController_Get_Enhanced.vi"("PhoenixMotorControlDevRef"=w586) -> ("PhoenixMotorControlDevRef"=w587:T10)  [unwired: 11 in, 3 out]
                n434 = call "CTRE_Phoenix_MotorControl_Set.vi"("error in (no error)"=w582, "Output"=w562, "Control Mode"=w581, "PhoenixMotorControlDevRef"=w578) -> ()  [unwired: 6 in, 2 out]
                n435 = call "CTRE_Phoenix_MotorControl_Set.vi"("error in (no error)"=w583, "Output"=w562, "Control Mode"=w584, "PhoenixMotorControlDevRef"=w587) -> ()  [unwired: 6 in, 2 out]
                n436 = call "Elapsed Time12"("Time Target (s)"=3.0, "Set Start Time (s)"=0.0) -> ("Time has Elapsed"=w560:bool)  [unwired: 10 in, 7 out]
                n437 = local read "speed"() -> (w572:dbl)
                n438 = call "CTRE_Phoenix_MotorControl_RefNumRegistryGet.vi"("refnum name"="Drive3") -> ("PhoenixMotorControlDevRef"=w594:T10)  [unwired: 9 in, 1 out]
                n439 = call "CTRE_Phoenix_MotorControl_RefNumRegistryGet.vi"("refnum name"="Drive2") -> ("PhoenixMotorControlDevRef"=w595:T10)  [unwired: 9 in, 1 out]
                n440 = call "CTRE_Phoenix_MotorControl_RefNumRegistryGet.vi"("refnum name"="Drive1") -> ("PhoenixMotorControlDevRef"=w596:T10)  [unwired: 9 in, 1 out]
                n441 = call "CTRE_Phoenix_MotorControl_RefNumRegistryGet.vi"("refnum name"="Drive0") -> ("PhoenixMotorControlDevRef"=w597:T10)  [unwired: 9 in, 1 out]
                n442 = case shown="True" w560 {
                  frame False {
                  }
                  frame True {
                    n443 = local write "speed"(0.0 ("speed")) -> ()
                    n444 = local write "stopped"(TRUE ("stopped")) -> ()
                  }
                }
                n445 = call <vilib>:"WPI_MotorControlSetOutput.vi"("Output"=w572, "MotorControlDevRef"=w594) -> ()  [unwired: 7 in, 3 out]
                n446 = call <vilib>:"WPI_MotorControlSetOutput.vi"("Output"=w572, "MotorControlDevRef"=w595) -> ()  [unwired: 7 in, 3 out]
                n447 = call <vilib>:"WPI_MotorControlSetOutput.vi"("Output"=w572, "MotorControlDevRef"=w596) -> ()  [unwired: 7 in, 3 out]
                n448 = call <vilib>:"WPI_MotorControlSetOutput.vi"("Output"=w572, "MotorControlDevRef"=w597) -> ()  [unwired: 7 in, 3 out]
              }
              n449 = while {
                shift-right: [w608] -> w552
                shift-left: w551 -> [w607]
                stop <- w604 stop-if-true
                # "Runs loop for about 116 days"
                # "Actual Auton"
                n450 = local read "stopped"() -> (w603:bool)
                n451 = case shown="True" w603 {
                  tunnel: [w610 w651] -> w608
                  tunnel: w607 -> [w609 w651]
                  frame False {
                    # "Auton 1: Basic Switch"
                    n452 = stacked-sequence {
                      tunnel: [w612 _ _] -> w610
                      tunnel: w609 -> [w611 _ _]
                      frame #0 {
                        n453 = while {
                          tunnel: [w623] -> w612
                          tunnel: w611 -> [w618]
                          stop <- w613 stop-if-true
                          # "Stops loop"
                          n454 = call <vilib>:"WPI_SerialPortGetBytesReceived.vi"("SerialPortRef"=w618) -> ("Bytes at Port"=w626:u32, "SerialPortRef"=w624:T19)  [unwired: 8 in, 1 out]
                          n455 = Greater Than 0?(x=w626) -> (x > 0?=w625:bool)
                          n456 = case shown="True" w625 {
                            tunnel: w626 -> [_ w633]
                            tunnel: w624 -> [w627 w632]
                            tunnel: [w627 w628] -> w623
                            frame False {
                            }
                            frame True {
                              # "Reads some stuff if we get some stuff"
                              n457 = local read "Text"() -> (w630:string)
                              n458 = call <vilib>:"WPI_SerialPortRead.vi"("Num Bytes to Read"=w633, "SerialPortRef"=w632) -> ("Buffer"=w629:string, "SerialPortRef"=w628:T19)  [unwired: 7 in, 1 out]
                              n459 = Concatenate Strings(w630, w629) -> (w631:string)
                              n460 = local write "Text"(w631) -> ()
                              n461 = local write "Current Reading"(w629) -> ()
                            }
                          }
                          n462 = local read "Text"() -> (w622:string)
                          n463 = Match Pattern(string=w622, regular expression="\\n") -> (offset past match=w620:i32)  [unwired: 1 in, 3 out]
                          n464 = Greater?(x=w620, y=-1) -> (0:w614:bool)
                          n465 = call "Elapsed Time9"("Time Target (s)"=3.0, "Set Start Time (s)"=0.0) -> ("Time has Elapsed"=w615:bool)  [unwired: 10 in, 7 out]
                          n466 = Or(x=w615, y=w614) -> (x .or. y?=w613:bool)
                        }
                      }
                      frame #1 {
                        # "Gives X (Left and Right) and Z (Distance)"
                        n467 = local read "Text"() -> (w639:string)
                        n468 = Match Pattern(string=w639, regular expression=",") -> (after substring=w637:string)  [unwired: 1 in, 3 out]
                        n469 = Match Pattern(string=w637, regular expression=",") -> (before substring=w635:string)  [unwired: 1 in, 3 out]
                        n470 = Decimal String To Number(string=w635) -> (number=w634:i32)  [unwired: 2 in, 1 out]
                        n471 = local write "x"(w634) -> ()
                      }
                      frame #2 {
                        # "Gives Direction to go!"
                        n472 = local read "x"() -> (w641:dbl)
                        n473 = Greater Than 0?(x=w641) -> (x > 0?=w640:bool)
                        n474 = local write "Text"("") -> ()
                        n475 = case shown="True" w640 {
                          frame False {
                          }
                          frame True {
                            n476 = local read "x"() -> (w647:dbl)
                            n477 = Divide(x=w647, y=320.0) -> (x/y=w646:dbl)
                            n478 = Multiply(x=w646, y=1800.0) -> (x*y=w648:dbl)
                            n479 = Subtract(x=900.0, y=w648) -> (x-y=w649:dbl)
                            n480 = local write "Direction"(w649) -> ()
                          }
                        }
                      }
                    }
                  }
                  frame True {
                    n481 = local read "CoolDown"() -> (w650:bool)
                    n482 = case shown="False" w650 {
                      frame False {
                        n483 = stacked-sequence {
                          frame #0 {
                            w652 = 1.0
                            n484 = call "CTRE_Phoenix_MotorControl_RefNumRegistryGet.vi"("refnum name"="Intake1") -> ("PhoenixMotorControlDevRef"=w653:T10)  [unwired: 9 in, 1 out]
                            n485 = call "CTRE_Phoenix_MotorControl_RefNumRegistryGet.vi"("refnum name"="Intake2") -> ("PhoenixMotorControlDevRef"=w656:T10)  [unwired: 9 in, 1 out]
                            n486 = Negate(x=w652) -> (-x=w657:dbl)
                            n487 = call <vilib>:"WPI_MotorControlSetOutput.vi"("Output"=w652, "MotorControlDevRef"=w656) -> ()  [unwired: 7 in, 3 out]
                            n488 = call <vilib>:"WPI_MotorControlSetOutput.vi"("Output"=w657, "MotorControlDevRef"=w653) -> ()  [unwired: 7 in, 3 out]
                            n489 = local write "Direction"(0.0 ("Direction")) -> ()
                            n490 = local write "speed"(0.0 ("speed")) -> ()
                            n491 = Wait (ms)(milliseconds to wait=u32 500) -> ()  [unwired: 1 out]
                          }
                          frame #1 {
                            n492 = while {
                              stop <- w667 stop-if-true
                              w661 = 0.0
                              n493 = call "CTRE_Phoenix_MotorControl_RefNumRegistryGet.vi"("refnum name"="Intake1") -> ("PhoenixMotorControlDevRef"=w662:T10)  [unwired: 9 in, 1 out]
                              n494 = call "CTRE_Phoenix_MotorControl_RefNumRegistryGet.vi"("refnum name"="Intake2") -> ("PhoenixMotorControlDevRef"=w665:T10)  [unwired: 9 in, 1 out]
                              n495 = local write "Direction"(2000.0 ("Direction")) -> ()
                              n496 = local write "speed"(0.4 ("speed")) -> ()
                              n497 = Negate(x=w661) -> (-x=w666:dbl)
                              n498 = call <vilib>:"WPI_MotorControlSetOutput.vi"("Output"=w661, "MotorControlDevRef"=w665) -> ()  [unwired: 7 in, 3 out]
                              n499 = call <vilib>:"WPI_MotorControlSetOutput.vi"("Output"=w666, "MotorControlDevRef"=w662) -> ()  [unwired: 7 in, 3 out]
                              n500 = call "Elapsed Time10"("Time Target (s)"=1.5, "Set Start Time (s)"=0.0) -> ("Time has Elapsed"=w667:bool)  [unwired: 10 in, 7 out]
                            }
                          }
                          frame #2 {
                            n501 = while {
                              stop <- w672 stop-if-true
                              n502 = local read "Switch"() -> (w677:bool)
                              n503 = local read "ElevatorDown"() -> (w679:dbl)
                              n504 = Select(t=-1000.0, s=w677, f=1000.0) -> (s? t:f=w678:dbl)
                              n505 = local write "Direction"(w678) -> ()
                              n506 = local write "speed"(0.4 ("speed")) -> ()
                              n507 = local write "ElevatePos"(w679) -> ()
                              n508 = call "Elapsed Time13"("Time Target (s)"=1.0, "Set Start Time (s)"=0.0) -> ("Time has Elapsed"=w672:bool)  [unwired: 10 in, 7 out]
                            }
                          }
                          frame #3 {
                            n509 = while {
                              stop <- w685 stop-if-true
                              n510 = call <vilib>:"WPI_SolenoidRefNum Registry Get.vi"("refnum name"="Open/Close") -> ("SolenoidDevRef"=w683:T20)  [unwired: 9 in, 1 out]
                              n511 = call-poly <vilib>:"WPI_SolenoidSet.vi"("Value"=TRUE, "SolenoidDevRef"=w683) -> ()  [unwired: 8 in, 2 out]
                              n512 = call "Elapsed Time16"("Time Target (s)"=1.5, "Set Start Time (s)"=0.0) -> ("Time has Elapsed"=w685:bool)  [unwired: 10 in, 7 out]
                              n513 = local write "Direction"(0.0 ("Direction")) -> ()
                              n514 = local write "speed"(0.4 ("speed")) -> ()
                            }
                          }
                          frame #4 {
                            n515 = while {
                              stop <- w693 stop-if-true
                              n516 = call <vilib>:"WPI_SolenoidRefNum Registry Get.vi"("refnum name"="Open/Close") -> ("SolenoidDevRef"=w691:T20)  [unwired: 9 in, 1 out]
                              n517 = call-poly <vilib>:"WPI_SolenoidSet.vi"("Value"=FALSE, "SolenoidDevRef"=w691) -> ()  [unwired: 8 in, 2 out]
                              n518 = call "Elapsed Time17"("Time Target (s)"=1.5, "Set Start Time (s)"=0.0) -> ("Time has Elapsed"=w693:bool)  [unwired: 10 in, 7 out]
                              n519 = local write "Direction"(0.0 ("Direction")) -> ()
                              n520 = local write "speed"(-0.4 ("speed")) -> ()
                            }
                          }
                          frame #5 {
                            n521 = while {
                              stop <- w702 stop-if-true
                              n522 = local read "ElevatorSwitch"() -> (w698:dbl)
                              n523 = local read "Switch"() -> (w701:bool)
                              n524 = local write "ElevatePos"(w698) -> ()
                              n525 = Select(t=1000.0, s=w701, f=-1000.0) -> (s? t:f=w697:dbl)
                              n526 = local write "Direction"(w697) -> ()
                              n527 = call "Elapsed Time18"("Time Target (s)"=1.0, "Set Start Time (s)"=0.0) -> ("Time has Elapsed"=w702:bool)  [unwired: 10 in, 7 out]
                              n528 = local write "speed"(0.4 ("speed")) -> ()
                            }
                          }
                          frame #6 {
                            w711 = 1.0
                            n529 = call "CTRE_Phoenix_MotorControl_RefNumRegistryGet.vi"("refnum name"="Intake1") -> ("PhoenixMotorControlDevRef"=w712:T10)  [unwired: 9 in, 1 out]
                            n530 = call "CTRE_Phoenix_MotorControl_RefNumRegistryGet.vi"("refnum name"="Intake2") -> ("PhoenixMotorControlDevRef"=w713:T10)  [unwired: 9 in, 1 out]
                            n531 = Negate(x=w711) -> (-x=w714:dbl)
                            n532 = call <vilib>:"WPI_MotorControlSetOutput.vi"("Output"=w711, "MotorControlDevRef"=w713) -> ()  [unwired: 7 in, 3 out]
                            n533 = call <vilib>:"WPI_MotorControlSetOutput.vi"("Output"=w714, "MotorControlDevRef"=w712) -> ()  [unwired: 7 in, 3 out]
                            n534 = local write "Direction"(0.0 ("Direction")) -> ()
                            n535 = local write "speed"(0.0 ("speed")) -> ()
                            n536 = Wait (ms)(milliseconds to wait=u32 500) -> ()  [unwired: 1 out]
                          }
                          frame #7 {
                            w717 = 0.0
                            n537 = call "CTRE_Phoenix_MotorControl_RefNumRegistryGet.vi"("refnum name"="Intake1") -> ("PhoenixMotorControlDevRef"=w718:T10)  [unwired: 9 in, 1 out]
                            n538 = call "CTRE_Phoenix_MotorControl_RefNumRegistryGet.vi"("refnum name"="Intake2") -> ("PhoenixMotorControlDevRef"=w719:T10)  [unwired: 9 in, 1 out]
                            n539 = Negate(x=w717) -> (-x=w720:dbl)
                            n540 = call <vilib>:"WPI_MotorControlSetOutput.vi"("Output"=w717, "MotorControlDevRef"=w719) -> ()  [unwired: 7 in, 3 out]
                            n541 = call <vilib>:"WPI_MotorControlSetOutput.vi"("Output"=w720, "MotorControlDevRef"=w718) -> ()  [unwired: 7 in, 3 out]
                            n542 = local write "Direction"(0.0 ("Direction")) -> ()
                            n543 = local write "speed"(-0.4 ("speed")) -> ()
                            n544 = Wait (ms)(milliseconds to wait=u32 1500) -> ()  [unwired: 1 out]
                          }
                          frame #8 {
                            n545 = local read "ElevatorDown"() -> (w725:dbl)
                            n546 = local write "CoolDown"(TRUE ("CoolDown")) -> ()
                            n547 = local write "ElevatePos"(w725) -> ()
                            n548 = local write "Direction"(0.0 ("Direction")) -> ()
                            n549 = local write "speed"(0.0 ("speed")) -> ()
                          }
                        }
                      }
                      frame True {
                      }
                    }
                  }
                }
                n550 = call "Elapsed Time11"("Time Target (s)"=14.0, "Set Start Time (s)"=0.0) -> ("Time has Elapsed"=w604:bool)  [unwired: 10 in, 7 out]
              }
              n551 = call <vilib>:"WPI_SerialPortClose.vi"("SerialPortRef"=w552) -> ()  [unwired: 10 in, 1 out]
            }
          }
        }
        frame -10 {
          n552 = stacked-sequence {
            frame #0 {
              n553 = Wait (ms)(milliseconds to wait=u32 750) -> ()  [unwired: 1 out]
            }
            frame #1 {
              n554 = while {
                stop <- w743 stop-if-true
                w730 = T6 1 items=["PercentOutput"=0, "Position"=1, "Velocity"=2, "Current"=3, "Follower"=5, "MotionProfile"=6, "MotionMagic"=7, "MotionMagicArc"=8, "MotionProfileArc"=10, "Disabled"=15] ("Control Mode")
                w746 = 0.4
                w748 = T6 1 items=["PercentOutput"=0, "Position"=1, "Velocity"=2, "Current"=3, "Follower"=5, "MotionProfile"=6, "MotionMagic"=7, "MotionMagicArc"=8, "MotionProfileArc"=10, "Disabled"=15] ("Control Mode")
                w755 = T6 1 items=["PercentOutput"=0, "Position"=1, "Velocity"=2, "Current"=3, "Follower"=5, "MotionProfile"=6, "MotionMagic"=7, "MotionMagicArc"=8, "MotionProfileArc"=10, "Disabled"=15] ("Control Mode")
                w758 = T6 1 items=["PercentOutput"=0, "Position"=1, "Velocity"=2, "Current"=3, "Follower"=5, "MotionProfile"=6, "MotionMagic"=7, "MotionMagicArc"=8, "MotionProfileArc"=10, "Disabled"=15] ("Control Mode")
                w772 = T6 1 items=["PercentOutput"=0, "Position"=1, "Velocity"=2, "Current"=3, "Follower"=5, "MotionProfile"=6, "MotionMagic"=7, "MotionMagicArc"=8, "MotionProfileArc"=10, "Disabled"=15] ("Control Mode")
                # "Turns and Moves the robot based on calculations"
                n555 = call <vilib>:"WPI_GyroRefNum Registry Get.vi"("refnum name"="Gyro") -> ("GyroDevRef"=w742:T7)  [unwired: 9 in, 1 out]
                n556 = call "CTRE_Phoenix_MotorControl_RefNumRegistryGet.vi"("refnum name"="Turn0") -> ("error out"=w747:errorcluster, "PhoenixMotorControlDevRef"=w750:T10)  [unwired: 9 in]
                n557 = call <vilib>:"WPI_GyroGetAngle.vi"("GyroDevRef"=w742) -> ("Angle"=w738:dbl)  [unwired: 6 in, 4 out]
                n558 = call "CTRE_Phoenix_MotorControl_RefNumRegistryGet.vi"("refnum name"="Turn1") -> ("error out"=w773:errorcluster, "PhoenixMotorControlDevRef"=w763:T10)  [unwired: 9 in]
                n559 = call-poly "CTRE_Phoenix_MotorController_Get_Enhanced.vi"("PhoenixMotorControlDevRef"=w750) -> ("PhoenixMotorControlDevRef"=w751:T10)  [unwired: 11 in, 3 out]
                n560 = global read "Robot Global Data.vi" "Gyro Centre"() -> (w739:dbl)
                n561 = call-poly "CTRE_Phoenix_MotorController_Get_Enhanced.vi"("PhoenixMotorControlDevRef"=w763) -> ("PhoenixMotorControlDevRef"=w762:T10)  [unwired: 11 in, 3 out]
                n562 = Subtract(x=w738, y=w739) -> (x-y=w740:dbl)
                n563 = Divide(x=w740, y=360.0) -> (x/y=w741:dbl)
                n564 = Multiply(x=w741, y=4096.0) -> (x*y=w734:dbl)
                n565 = call "CTRE_Phoenix_MotorControl_Set.vi"("error in (no error)"=w747, "Output"=w734, "Control Mode"=w748, "PhoenixMotorControlDevRef"=w751) -> ()  [unwired: 6 in, 2 out]
                n566 = call "CTRE_Phoenix_MotorControl_Set.vi"("error in (no error)"=w773, "Output"=w734, "Control Mode"=w772, "PhoenixMotorControlDevRef"=w762) -> ()  [unwired: 6 in, 2 out]
                n567 = call "CTRE_Phoenix_MotorControl_RefNumRegistryGet.vi"("refnum name"="Turn3") -> ("error out"=w756:errorcluster, "PhoenixMotorControlDevRef"=w753:T10)  [unwired: 9 in]
                n568 = call "CTRE_Phoenix_MotorControl_RefNumRegistryGet.vi"("refnum name"="Turn2") -> ("error out"=w757:errorcluster, "PhoenixMotorControlDevRef"=w760:T10)  [unwired: 9 in]
                n569 = local read "ElevatorPyramid"() -> (w729:dbl)
                n570 = call "CTRE_Phoenix_MotorControl_RefNumRegistryGet.vi"("refnum name"="Elevator") -> ("PhoenixMotorControlDevRef"=w731:T10)  [unwired: 9 in, 1 out]
                n571 = call-poly "CTRE_Phoenix_MotorController_Get_Enhanced.vi"("PhoenixMotorControlDevRef"=w753) -> ("PhoenixMotorControlDevRef"=w752:T10)  [unwired: 11 in, 3 out]
                n572 = call-poly "CTRE_Phoenix_MotorController_Get_Enhanced.vi"("PhoenixMotorControlDevRef"=w760) -> ("PhoenixMotorControlDevRef"=w761:T10)  [unwired: 11 in, 3 out]
                n573 = call "CTRE_Phoenix_MotorControl_Set.vi"("Output"=w729, "Control Mode"=w730, "PhoenixMotorControlDevRef"=w731) -> ()  [unwired: 7 in, 2 out]
                n574 = call "CTRE_Phoenix_MotorControl_Set.vi"("error in (no error)"=w756, "Output"=w734, "Control Mode"=w755, "PhoenixMotorControlDevRef"=w752) -> ()  [unwired: 6 in, 2 out]
                n575 = call "CTRE_Phoenix_MotorControl_Set.vi"("error in (no error)"=w757, "Output"=w734, "Control Mode"=w758, "PhoenixMotorControlDevRef"=w761) -> ()  [unwired: 6 in, 2 out]
                n576 = call "Elapsed Time4"("Time Target (s)"=3.5, "Set Start Time (s)"=0.0) -> ("Time has Elapsed"=w743:bool)  [unwired: 10 in, 7 out]
                n577 = call "CTRE_Phoenix_MotorControl_RefNumRegistryGet.vi"("refnum name"="Drive3") -> ("PhoenixMotorControlDevRef"=w768:T10)  [unwired: 9 in, 1 out]
                n578 = call "CTRE_Phoenix_MotorControl_RefNumRegistryGet.vi"("refnum name"="Drive2") -> ("PhoenixMotorControlDevRef"=w769:T10)  [unwired: 9 in, 1 out]
                n579 = call "CTRE_Phoenix_MotorControl_RefNumRegistryGet.vi"("refnum name"="Drive1") -> ("PhoenixMotorControlDevRef"=w770:T10)  [unwired: 9 in, 1 out]
                n580 = call "CTRE_Phoenix_MotorControl_RefNumRegistryGet.vi"("refnum name"="Drive0") -> ("PhoenixMotorControlDevRef"=w771:T10)  [unwired: 9 in, 1 out]
                n581 = call <vilib>:"WPI_MotorControlSetOutput.vi"("Output"=w746, "MotorControlDevRef"=w768) -> ()  [unwired: 7 in, 3 out]
                n582 = call <vilib>:"WPI_MotorControlSetOutput.vi"("Output"=w746, "MotorControlDevRef"=w769) -> ()  [unwired: 7 in, 3 out]
                n583 = call <vilib>:"WPI_MotorControlSetOutput.vi"("Output"=w746, "MotorControlDevRef"=w770) -> ()  [unwired: 7 in, 3 out]
                n584 = call <vilib>:"WPI_MotorControlSetOutput.vi"("Output"=w746, "MotorControlDevRef"=w771) -> ()  [unwired: 7 in, 3 out]
              }
            }
            frame #2 {
              w778 = 0.0
              n585 = call "CTRE_Phoenix_MotorControl_RefNumRegistryGet.vi"("refnum name"="Drive3") -> ("PhoenixMotorControlDevRef"=w779:T10)  [unwired: 9 in, 1 out]
              n586 = call "CTRE_Phoenix_MotorControl_RefNumRegistryGet.vi"("refnum name"="Drive2") -> ("PhoenixMotorControlDevRef"=w780:T10)  [unwired: 9 in, 1 out]
              n587 = call "CTRE_Phoenix_MotorControl_RefNumRegistryGet.vi"("refnum name"="Drive1") -> ("PhoenixMotorControlDevRef"=w781:T10)  [unwired: 9 in, 1 out]
              n588 = call "CTRE_Phoenix_MotorControl_RefNumRegistryGet.vi"("refnum name"="Drive0") -> ("PhoenixMotorControlDevRef"=w782:T10)  [unwired: 9 in, 1 out]
              n589 = call <vilib>:"WPI_MotorControlSetOutput.vi"("Output"=w778, "MotorControlDevRef"=w779) -> ()  [unwired: 7 in, 3 out]
              n590 = call <vilib>:"WPI_MotorControlSetOutput.vi"("Output"=w778, "MotorControlDevRef"=w780) -> ()  [unwired: 7 in, 3 out]
              n591 = call <vilib>:"WPI_MotorControlSetOutput.vi"("Output"=w778, "MotorControlDevRef"=w781) -> ()  [unwired: 7 in, 3 out]
              n592 = call <vilib>:"WPI_MotorControlSetOutput.vi"("Output"=w778, "MotorControlDevRef"=w782) -> ()  [unwired: 7 in, 3 out]
            }
          }
        }
        frame 0 {
        }
        frame 6 {
          # "Left 2 Scale/Switch"
          n593 = while {
            stop <- FALSE stop-if-true
            w958 = T6 7 items=["PercentOutput"=0, "Position"=1, "Velocity"=2, "Current"=3, "Follower"=5, "MotionProfile"=6, "MotionMagic"=7, "MotionMagicArc"=8, "MotionProfileArc"=10, "Disabled"=15] ("Control Mode")
            w990 = T6 1 items=["PercentOutput"=0, "Position"=1, "Velocity"=2, "Current"=3, "Follower"=5, "MotionProfile"=6, "MotionMagic"=7, "MotionMagicArc"=8, "MotionProfileArc"=10, "Disabled"=15] ("Control Mode")
            w988 = T6 1 items=["PercentOutput"=0, "Position"=1, "Velocity"=2, "Current"=3, "Follower"=5, "MotionProfile"=6, "MotionMagic"=7, "MotionMagicArc"=8, "MotionProfileArc"=10, "Disabled"=15] ("Control Mode")
            w986 = T6 1 items=["PercentOutput"=0, "Position"=1, "Velocity"=2, "Current"=3, "Follower"=5, "MotionProfile"=6, "MotionMagic"=7, "MotionMagicArc"=8, "MotionProfileArc"=10, "Disabled"=15] ("Control Mode")
            w980 = T6 1 items=["PercentOutput"=0, "Position"=1, "Velocity"=2, "Current"=3, "Follower"=5, "MotionProfile"=6, "MotionMagic"=7, "MotionMagicArc"=8, "MotionProfileArc"=10, "Disabled"=15] ("Control Mode")
            # "Turns and Moves the robot based on calculations"
            n594 = local read "ElevatePos"() -> (w960:dbl)
            n595 = call <vilib>:"WPI_GyroRefNum Registry Get.vi"("refnum name"="Gyro") -> ("GyroDevRef"=w972:T7)  [unwired: 9 in, 1 out]
            n596 = call "CTRE_Phoenix_MotorControl_RefNumRegistryGet.vi"("refnum name"="Elevator") -> ("PhoenixMotorControlDevRef"=w959:T10)  [unwired: 9 in, 1 out]
            n597 = call <vilib>:"WPI_GyroGetAngle.vi"("GyroDevRef"=w972) -> ("Angle"=w977:dbl)  [unwired: 6 in, 4 out]
            n598 = call "CTRE_Phoenix_MotorControl_Set.vi"("Output"=w960, "Control Mode"=w958, "PhoenixMotorControlDevRef"=w959) -> ()  [unwired: 7 in, 2 out]
            n599 = global read "Robot Global Data.vi" "Gyro Centre"() -> (w976:dbl)
            n600 = Subtract(x=w977, y=w976) -> (x-y=w975:dbl)
            n601 = Divide(x=w975, y=360.0) -> (x/y=w973:dbl)
            n602 = Multiply(x=w973, y=4096.0) -> (x*y=w962:dbl)
            n603 = call "CTRE_Phoenix_MotorControl_RefNumRegistryGet.vi"("refnum name"="Turn0") -> ("error out"=w991:errorcluster, "PhoenixMotorControlDevRef"=w992:T10)  [unwired: 9 in]
            n604 = call "CTRE_Phoenix_MotorControl_RefNumRegistryGet.vi"("refnum name"="Turn1") -> ("error out"=w1006:errorcluster, "PhoenixMotorControlDevRef"=w1001:T10)  [unwired: 9 in]
            n605 = local read "Direction"() -> (w968:dbl)
            n606 = local read "Direction 1"() -> (w963:dbl)
            n607 = call-poly "CTRE_Phoenix_MotorController_Get_Enhanced.vi"("PhoenixMotorControlDevRef"=w992) -> ("PhoenixMotorControlDevRef"=w993:T10)  [unwired: 11 in, 3 out]
            n608 = call-poly "CTRE_Phoenix_MotorController_Get_Enhanced.vi"("PhoenixMotorControlDevRef"=w1001) -> ("PhoenixMotorControlDevRef"=w1000:T10)  [unwired: 11 in, 3 out]
            n609 = Add(x=w962, y=w968) -> (x+y=w967:dbl)
            n610 = Add(x=w962, y=w963) -> (x+y=w961:dbl)
            n611 = call "CTRE_Phoenix_MotorControl_Set.vi"("error in (no error)"=w991, "Output"=w967, "Control Mode"=w990, "PhoenixMotorControlDevRef"=w993) -> ()  [unwired: 6 in, 2 out]
            n612 = call "CTRE_Phoenix_MotorControl_Set.vi"("error in (no error)"=w1006, "Output"=w961, "Control Mode"=w980, "PhoenixMotorControlDevRef"=w1000) -> ()  [unwired: 6 in, 2 out]
            n613 = call "CTRE_Phoenix_MotorControl_RefNumRegistryGet.vi"("refnum name"="Turn3") -> ("error out"=w996:errorcluster, "PhoenixMotorControlDevRef"=w995:T10)  [unwired: 9 in]
            n614 = call "CTRE_Phoenix_MotorControl_RefNumRegistryGet.vi"("refnum name"="Turn2") -> ("error out"=w997:errorcluster, "PhoenixMotorControlDevRef"=w998:T10)  [unwired: 9 in]
            n615 = local read "Direction 2"() -> (w966:dbl)
            n616 = local read "Direction 3"() -> (w970:dbl)
            n617 = call-poly "CTRE_Phoenix_MotorController_Get_Enhanced.vi"("PhoenixMotorControlDevRef"=w995) -> ("PhoenixMotorControlDevRef"=w994:T10)  [unwired: 11 in, 3 out]
            n618 = call-poly "CTRE_Phoenix_MotorController_Get_Enhanced.vi"("PhoenixMotorControlDevRef"=w998) -> ("PhoenixMotorControlDevRef"=w999:T10)  [unwired: 11 in, 3 out]
            n619 = Add(x=w966, y=w962) -> (x+y=w965:dbl)
            n620 = Add(x=w970, y=w962) -> (x+y=w969:dbl)
            n621 = call "CTRE_Phoenix_MotorControl_Set.vi"("error in (no error)"=w996, "Output"=w969, "Control Mode"=w988, "PhoenixMotorControlDevRef"=w994) -> ()  [unwired: 6 in, 2 out]
            n622 = call "CTRE_Phoenix_MotorControl_Set.vi"("error in (no error)"=w997, "Output"=w965, "Control Mode"=w986, "PhoenixMotorControlDevRef"=w999) -> ()  [unwired: 6 in, 2 out]
            n623 = local read "speed"() -> (w1007:dbl)
            n624 = call "CTRE_Phoenix_MotorControl_RefNumRegistryGet.vi"("refnum name"="Drive3") -> ("PhoenixMotorControlDevRef"=w1002:T10)  [unwired: 9 in, 1 out]
            n625 = call "CTRE_Phoenix_MotorControl_RefNumRegistryGet.vi"("refnum name"="Drive2") -> ("PhoenixMotorControlDevRef"=w1003:T10)  [unwired: 9 in, 1 out]
            n626 = call "CTRE_Phoenix_MotorControl_RefNumRegistryGet.vi"("refnum name"="Drive1") -> ("PhoenixMotorControlDevRef"=w1004:T10)  [unwired: 9 in, 1 out]
            n627 = call "CTRE_Phoenix_MotorControl_RefNumRegistryGet.vi"("refnum name"="Drive0") -> ("PhoenixMotorControlDevRef"=w1005:T10)  [unwired: 9 in, 1 out]
            n628 = call <vilib>:"WPI_MotorControlSetOutput.vi"("Output"=w1007, "MotorControlDevRef"=w1002) -> ()  [unwired: 7 in, 3 out]
            n629 = call <vilib>:"WPI_MotorControlSetOutput.vi"("Output"=w1007, "MotorControlDevRef"=w1003) -> ()  [unwired: 7 in, 3 out]
            n630 = call <vilib>:"WPI_MotorControlSetOutput.vi"("Output"=w1007, "MotorControlDevRef"=w1004) -> ()  [unwired: 7 in, 3 out]
            n631 = call <vilib>:"WPI_MotorControlSetOutput.vi"("Output"=w1007, "MotorControlDevRef"=w1005) -> ()  [unwired: 7 in, 3 out]
          }
          n632 = stacked-sequence {
            frame #0 {
              w786 = -100.0 ("Direction")
              n633 = local write "speed"(0.8 ("speed")) -> ()
              n634 = local write "Direction 3"(w786) -> ()
              n635 = local write "Direction 1"(w786) -> ()
              n636 = local write "Direction 2"(w786) -> ()
              n637 = local write "Direction"(w786) -> ()
              n638 = Wait (ms)(milliseconds to wait=u32 1750) -> ()  [unwired: 1 out]
              n639 = local read "ElevatorPyramid"() -> (w783:dbl)
              n640 = local write "ElevatePos"(w783) -> ()
            }
            frame #1 {
              n641 = local read "Scale"() -> (w787:bool)
              n642 = case shown="True" w787 {
                frame False {
                  n643 = local read "ElevatorDown"() -> (w788:dbl)
                  n644 = local write "speed"(0.0 ("speed")) -> ()
                  n645 = local write "ElevatePos"(w788) -> ()
                }
                frame True {
                  # "2 Scale"
                  n646 = stacked-sequence {
                    frame #0 {
                      n647 = Wait (ms)(milliseconds to wait=u32 1000) -> ()  [unwired: 1 out]
                    }
                    frame #1 {
                      n648 = while {
                        stop <- w795 stop-if-true
                        n649 = call <vilib>:"WPI_GyroRefNum Registry Get.vi"("refnum name"="Gyro") -> ("GyroDevRef"=w820:T7)  [unwired: 9 in, 1 out]
                        n650 = call <vilib>:"WPI_GyroGetAngle.vi"("GyroDevRef"=w820) -> ("Angle"=w816:dbl)  [unwired: 6 in, 4 out]
                        n651 = global read "Robot Global Data.vi" "Gyro Centre"() -> (w817:dbl)
                        n652 = Subtract(x=w816, y=w817) -> (x-y=w806:dbl)
                        n653 = Quotient & Remainder(x=w806, y=360.0) -> (x-y*floor(x/y)=w804:dbl)  [unwired: 1 out]
                        n654 = Divide(x=w806, y=360.0) -> (x/y=w819:dbl)
                        n655 = Multiply(x=w819, y=4096.0) -> (x*y=w807:dbl)
                        n656 = Subtract(x=2500.0, y=w807) -> (x-y=w814:dbl)
                        n657 = Less Or Equal?(x=w804, y=60.0) -> (x <= y?=w801:bool)
                        n658 = Greater Or Equal?(x=w804, y=30.0) -> (x >= y?=w800:bool)
                        n659 = local write "Direction"(w814) -> ()
                        n660 = And(x=w801, y=w800) -> (x .and. y?=w791:bool)
                        n661 = Subtract(x=1500.0, y=w807) -> (x-y=w813:dbl)
                        n662 = case shown="False" w791 {
                          frame False {
                            n663 = local write "speed"(0.3 ("speed")) -> ()
                          }
                          frame True {
                            n664 = local write "speed"(0.0 ("speed")) -> ()
                          }
                        }
                        n665 = local write "Direction 1"(w813) -> ()
                        n666 = local read "ElevatorScale"() -> (w799:dbl)
                        n667 = Subtract(x=500.0, y=w807) -> (x-y=w810:dbl)
                        n668 = local write "Direction 2"(w810) -> ()
                        n669 = local write "ElevatePos"(w799) -> ()
                        n670 = call "CTRE_Phoenix_MotorControl_RefNumRegistryGet.vi"("refnum name"="Elevator") -> ("error out"=w796:errorcluster, "PhoenixMotorControlDevRef"=w797:T10)  [unwired: 9 in]
                        n671 = call-poly "CTRE_Phoenix_MotorController_Get_Enhanced.vi"("PhoenixMotorControlDevRef"=w797, "error in"=w796) -> ("Pulse Width Position"=w794:i32)  [unwired: 8 in, 5 out]
                        n672 = Subtract(x=3500.0, y=w807) -> (x-y=w809:dbl)
                        n673 = local write "Direction 3"(w809) -> ()
                        n674 = Less?(x=w794, y=-30500) -> (x < y?=w792:bool)
                        n675 = And(x=w792, y=w791) -> (x .and. y?=w795:bool)
                      }
                    }
                    frame #2 {
                      w825 = T6 1 items=["PercentOutput"=0, "Position"=1, "Velocity"=2, "Current"=3, "Follower"=5, "MotionProfile"=6, "MotionMagic"=7, "MotionMagicArc"=8, "MotionProfileArc"=10, "Disabled"=15] ("Control Mode")
                      w830 = 0.0 ("Direction")
                      n676 = call "CTRE_Phoenix_MotorControl_RefNumRegistryGet.vi"("refnum name"="IntakeUp") -> ("PhoenixMotorControlDevRef"=w828:T10)  [unwired: 9 in, 1 out]
                      n677 = call "CTRE_Phoenix_MotorControl_Set.vi"("Output"=-2000.0, "Control Mode"=w825, "PhoenixMotorControlDevRef"=w828) -> ()  [unwired: 7 in, 2 out]
                      n678 = local write "Direction 3"(w830) -> ()
                      n679 = local write "Direction 2"(w830) -> ()
                      n680 = local write "Direction 1"(w830) -> ()
                      n681 = local write "speed"(0.4 ("speed")) -> ()
                      n682 = local write "Direction"(w830) -> ()
                      n683 = Wait (ms)(milliseconds to wait=u32 1250) -> ()  [unwired: 1 out]
                    }
                    frame #3 {
                      w836 = T6 0 items=["PercentOutput"=0, "Position"=1, "Velocity"=2, "Current"=3, "Follower"=5, "MotionProfile"=6, "MotionMagic"=7, "MotionMagicArc"=8, "MotionProfileArc"=10, "Disabled"=15] ("Control Mode")
                      w833 = T6 0 items=["PercentOutput"=0, "Position"=1, "Velocity"=2, "Current"=3, "Follower"=5, "MotionProfile"=6, "MotionMagic"=7, "MotionMagicArc"=8, "MotionProfileArc"=10, "Disabled"=15] ("Control Mode")
                      w843 = 0.0 ("Direction")
                      n684 = call "CTRE_Phoenix_MotorControl_RefNumRegistryGet.vi"("refnum name"="Intake1") -> ("error out"=w838:errorcluster, "PhoenixMotorControlDevRef"=w839:T10)  [unwired: 9 in]
                      n685 = call "CTRE_Phoenix_MotorControl_RefNumRegistryGet.vi"("refnum name"="Intake2") -> ("error out"=w841:errorcluster, "PhoenixMotorControlDevRef"=w840:T10)  [unwired: 9 in]
                      n686 = call "CTRE_Phoenix_MotorControl_Set.vi"("error in (no error)"=w838, "Output"=-1.0, "Control Mode"=w833, "PhoenixMotorControlDevRef"=w839) -> ()  [unwired: 6 in, 2 out]
                      n687 = call "CTRE_Phoenix_MotorControl_Set.vi"("error in (no error)"=w841, "Output"=1.0, "Control Mode"=w836, "PhoenixMotorControlDevRef"=w840) -> ()  [unwired: 6 in, 2 out]
                      n688 = local write "Direction 3"(w843) -> ()
                      n689 = local write "Direction 2"(w843) -> ()
                      n690 = local write "Direction 1"(w843) -> ()
                      n691 = local write "speed"(0.0 ("speed")) -> ()
                      n692 = local write "Direction"(w843) -> ()
                      n693 = Wait (ms)(milliseconds to wait=u32 1000) -> ()  [unwired: 1 out]
                    }
                    frame #4 {
                      w848 = T6 1 items=["PercentOutput"=0, "Position"=1, "Velocity"=2, "Current"=3, "Follower"=5, "MotionProfile"=6, "MotionMagic"=7, "MotionMagicArc"=8, "MotionProfileArc"=10, "Disabled"=15] ("Control Mode")
                      w854 = T6 0 items=["PercentOutput"=0, "Position"=1, "Velocity"=2, "Current"=3, "Follower"=5, "MotionProfile"=6, "MotionMagic"=7, "MotionMagicArc"=8, "MotionProfileArc"=10, "Disabled"=15] ("Control Mode")
                      w851 = T6 0 items=["PercentOutput"=0, "Position"=1, "Velocity"=2, "Current"=3, "Follower"=5, "MotionProfile"=6, "MotionMagic"=7, "MotionMagicArc"=8, "MotionProfileArc"=10, "Disabled"=15] ("Control Mode")
                      w860 = 2000.0 ("Direction")
                      n694 = call "CTRE_Phoenix_MotorControl_RefNumRegistryGet.vi"("refnum name"="IntakeUp") -> ("PhoenixMotorControlDevRef"=w845:T10)  [unwired: 9 in, 1 out]
                      n695 = local write "Direction 3"(w860) -> ()
                      n696 = local write "Direction 2"(w860) -> ()
                      n697 = local write "Direction 1"(w860) -> ()
                      n698 = local write "speed"(0.4 ("speed")) -> ()
                      n699 = local write "Direction"(w860) -> ()
                      n700 = call "CTRE_Phoenix_MotorControl_RefNumRegistryGet.vi"("refnum name"="Intake1") -> ("error out"=w855:errorcluster, "PhoenixMotorControlDevRef"=w856:T10)  [unwired: 9 in]
                      n701 = call "CTRE_Phoenix_MotorControl_RefNumRegistryGet.vi"("refnum name"="Intake2") -> ("error out"=w858:errorcluster, "PhoenixMotorControlDevRef"=w857:T10)  [unwired: 9 in]
                      n702 = call "CTRE_Phoenix_MotorControl_Set.vi"("Output"=-4500.0, "Control Mode"=w848, "PhoenixMotorControlDevRef"=w845) -> ()  [unwired: 7 in, 2 out]
                      n703 = call "CTRE_Phoenix_MotorControl_Set.vi"("error in (no error)"=w855, "Output"=0.0, "Control Mode"=w851, "PhoenixMotorControlDevRef"=w856) -> ()  [unwired: 6 in, 2 out]
                      n704 = call "CTRE_Phoenix_MotorControl_Set.vi"("error in (no error)"=w858, "Output"=0.0, "Control Mode"=w854, "PhoenixMotorControlDevRef"=w857) -> ()  [unwired: 6 in, 2 out]
                      n705 = Wait (ms)(milliseconds to wait=u32 1250) -> ()  [unwired: 1 out]
                    }
                    frame #5 {
                      n706 = while {
                        stop <- w867 stop-if-true
                        n707 = local read "ElevatorDown"() -> (w862:dbl)
                        n708 = call <vilib>:"WPI_GyroRefNum Registry Get.vi"("refnum name"="Gyro") -> ("GyroDevRef"=w891:T7)  [unwired: 9 in, 1 out]
                        n709 = call <vilib>:"WPI_GyroGetAngle.vi"("GyroDevRef"=w891) -> ("Angle"=w887:dbl)  [unwired: 6 in, 4 out]
                        n710 = global read "Robot Global Data.vi" "Gyro Centre"() -> (w888:dbl)
                        n711 = local write "ElevatePos"(w862) -> ()
                        n712 = Subtract(x=w887, y=w888) -> (x-y=w877:dbl)
                        n713 = Quotient & Remainder(x=w877, y=360.0) -> (x-y*floor(x/y)=w875:dbl)  [unwired: 1 out]
                        n714 = Divide(x=w877, y=360.0) -> (x/y=w890:dbl)
                        n715 = Multiply(x=w890, y=4096.0) -> (x*y=w878:dbl)
                        n716 = Subtract(x=2500.0, y=w878) -> (x-y=w885:dbl)
                        n717 = Less Or Equal?(x=w875, y=200.0) -> (x <= y?=w872:bool)
                        n718 = Greater Or Equal?(x=w875, y=160.0) -> (x >= y?=w871:bool)
                        n719 = local write "Direction"(w885) -> ()
                        n720 = And(x=w872, y=w871) -> (x .and. y?=w863:bool)
                        n721 = Subtract(x=1500.0, y=w878) -> (x-y=w884:dbl)
                        n722 = case shown="False" w863 {
                          frame False {
                            n723 = local write "speed"(0.3 ("speed")) -> ()
                          }
                          frame True {
                            n724 = local write "speed"(0.0 ("speed")) -> ()
                          }
                        }
                        n725 = local write "Direction 1"(w884) -> ()
                        n726 = Subtract(x=500.0, y=w878) -> (x-y=w881:dbl)
                        n727 = local write "Direction 2"(w881) -> ()
                        n728 = call "CTRE_Phoenix_MotorControl_RefNumRegistryGet.vi"("refnum name"="Elevator") -> ("error out"=w868:errorcluster, "PhoenixMotorControlDevRef"=w869:T10)  [unwired: 9 in]
                        n729 = call-poly "CTRE_Phoenix_MotorController_Get_Enhanced.vi"("PhoenixMotorControlDevRef"=w869, "error in"=w868) -> ("Pulse Width Position"=w866:i32)  [unwired: 8 in, 5 out]
                        n730 = Subtract(x=3500.0, y=w878) -> (x-y=w880:dbl)
                        n731 = local write "Direction 3"(w880) -> ()
                        n732 = Greater?(x=w866, y=-900) -> (0:w864:bool)
                        n733 = And(x=w864, y=w863) -> (x .and. y?=w867:bool)
                      }
                      n734 = while {
                        stop <- w901 stop-if-true
                        n735 = local read "ElevatorDown"() -> (w896:dbl)
                        n736 = call <vilib>:"WPI_GyroRefNum Registry Get.vi"("refnum name"="Gyro") -> ("GyroDevRef"=w925:T7)  [unwired: 9 in, 1 out]
                        n737 = call <vilib>:"WPI_GyroGetAngle.vi"("GyroDevRef"=w925) -> ("Angle"=w921:dbl)  [unwired: 6 in, 4 out]
                        n738 = global read "Robot Global Data.vi" "Gyro Centre"() -> (w922:dbl)
                        n739 = local write "ElevatePos"(w896) -> ()
                        n740 = Subtract(x=w921, y=w922) -> (x-y=w911:dbl)
                        n741 = Quotient & Remainder(x=w911, y=360.0) -> (x-y*floor(x/y)=w909:dbl)  [unwired: 1 out]
                        n742 = Divide(x=w911, y=360.0) -> (x/y=w924:dbl)
                        n743 = Multiply(x=w924, y=4096.0) -> (x*y=w912:dbl)
                        n744 = Subtract(x=2500.0, y=w912) -> (x-y=w919:dbl)
                        n745 = Less Or Equal?(x=w909, y=200.0) -> (x <= y?=w906:bool)
                        n746 = Greater Or Equal?(x=w909, y=160.0) -> (x >= y?=w905:bool)
                        n747 = local write "Direction"(w919) -> ()
                        n748 = And(x=w906, y=w905) -> (x .and. y?=w897:bool)
                        n749 = Subtract(x=1500.0, y=w912) -> (x-y=w918:dbl)
                        n750 = case shown="False" w897 {
                          frame False {
                            n751 = local write "speed"(0.3 ("speed")) -> ()
                          }
                          frame True {
                            n752 = local write "speed"(0.0 ("speed")) -> ()
                          }
                        }
                        n753 = local write "Direction 1"(w918) -> ()
                        n754 = Subtract(x=500.0, y=w912) -> (x-y=w915:dbl)
                        n755 = local write "Direction 2"(w915) -> ()
                        n756 = call "CTRE_Phoenix_MotorControl_RefNumRegistryGet.vi"("refnum name"="Elevator") -> ("error out"=w902:errorcluster, "PhoenixMotorControlDevRef"=w903:T10)  [unwired: 9 in]
                        n757 = call-poly "CTRE_Phoenix_MotorController_Get_Enhanced.vi"("PhoenixMotorControlDevRef"=w903, "error in"=w902) -> ("Pulse Width Position"=w900:i32)  [unwired: 8 in, 5 out]
                        n758 = Subtract(x=3500.0, y=w912) -> (x-y=w914:dbl)
                        n759 = local write "Direction 3"(w914) -> ()
                        n760 = Greater?(x=w900, y=-900) -> (0:w898:bool)
                        n761 = And(x=w898, y=w897) -> (x .and. y?=w901:bool)
                      }
                    }
                    frame #6 {
                      n762 = while {
                        stop <- w932 stop-if-true
                        w939 = T6 0 items=["PercentOutput"=0, "Position"=1, "Velocity"=2, "Current"=3, "Follower"=5, "MotionProfile"=6, "MotionMagic"=7, "MotionMagicArc"=8, "MotionProfileArc"=10, "Disabled"=15] ("Control Mode")
                        w936 = T6 0 items=["PercentOutput"=0, "Position"=1, "Velocity"=2, "Current"=3, "Follower"=5, "MotionProfile"=6, "MotionMagic"=7, "MotionMagicArc"=8, "MotionProfileArc"=10, "Disabled"=15] ("Control Mode")
                        w934 = 2048.0 ("Direction")
                        n763 = call "CTRE_Phoenix_MotorControl_RefNumRegistryGet.vi"("refnum name"="Intake1") -> ("error out"=w941:errorcluster, "PhoenixMotorControlDevRef"=w942:T10)  [unwired: 9 in]
                        n764 = call "CTRE_Phoenix_MotorControl_RefNumRegistryGet.vi"("refnum name"="Intake2") -> ("error out"=w944:errorcluster, "PhoenixMotorControlDevRef"=w943:T10)  [unwired: 9 in]
                        n765 = call "CTRE_Phoenix_MotorControl_Set.vi"("error in (no error)"=w941, "Output"=1.0, "Control Mode"=w936, "PhoenixMotorControlDevRef"=w942) -> ()  [unwired: 6 in, 2 out]
                        n766 = call "CTRE_Phoenix_MotorControl_Set.vi"("error in (no error)"=w944, "Output"=-1.0, "Control Mode"=w939, "PhoenixMotorControlDevRef"=w943) -> ()  [unwired: 6 in, 2 out]
                        n767 = local write "Direction 3"(w934) -> ()
                        n768 = call "Elapsed Time5"("Time Target (s)"=2.0, "Set Start Time (s)"=0.0) -> ("Time has Elapsed"=w932:bool)  [unwired: 10 in, 7 out]
                        n769 = local write "Direction 2"(w934) -> ()
                        n770 = local write "Direction 1"(w934) -> ()
                        n771 = local write "speed"(0.5 ("speed")) -> ()
                        n772 = local write "Direction"(w934) -> ()
                      }
                    }
                    frame #7 {
                      w951 = T6 0 items=["PercentOutput"=0, "Position"=1, "Velocity"=2, "Current"=3, "Follower"=5, "MotionProfile"=6, "MotionMagic"=7, "MotionMagicArc"=8, "MotionProfileArc"=10, "Disabled"=15] ("Control Mode")
                      w948 = T6 0 items=["PercentOutput"=0, "Position"=1, "Velocity"=2, "Current"=3, "Follower"=5, "MotionProfile"=6, "MotionMagic"=7, "MotionMagicArc"=8, "MotionProfileArc"=10, "Disabled"=15] ("Control Mode")
                      w946 = 2048.0 ("Direction")
                      n773 = call "CTRE_Phoenix_MotorControl_RefNumRegistryGet.vi"("refnum name"="Intake1") -> ("error out"=w953:errorcluster, "PhoenixMotorControlDevRef"=w954:T10)  [unwired: 9 in]
                      n774 = call "CTRE_Phoenix_MotorControl_RefNumRegistryGet.vi"("refnum name"="Intake2") -> ("error out"=w956:errorcluster, "PhoenixMotorControlDevRef"=w955:T10)  [unwired: 9 in]
                      n775 = call "CTRE_Phoenix_MotorControl_Set.vi"("error in (no error)"=w953, "Output"=0.0, "Control Mode"=w948, "PhoenixMotorControlDevRef"=w954) -> ()  [unwired: 6 in, 2 out]
                      n776 = call "CTRE_Phoenix_MotorControl_Set.vi"("error in (no error)"=w956, "Output"=0.0, "Control Mode"=w951, "PhoenixMotorControlDevRef"=w955) -> ()  [unwired: 6 in, 2 out]
                      n777 = local write "Direction 3"(w946) -> ()
                      n778 = local write "Direction 2"(w946) -> ()
                      n779 = local write "Direction 1"(w946) -> ()
                      n780 = local write "speed"(0.0 ("speed")) -> ()
                      n781 = local write "Direction"(w946) -> ()
                    }
                  }
                }
              }
            }
          }
        }
        frame -2 {
          # "Right Scale"
          n782 = while {
            stop <- FALSE stop-if-true
            w1091 = T6 7 items=["PercentOutput"=0, "Position"=1, "Velocity"=2, "Current"=3, "Follower"=5, "MotionProfile"=6, "MotionMagic"=7, "MotionMagicArc"=8, "MotionProfileArc"=10, "Disabled"=15] ("Control Mode")
            w1123 = T6 1 items=["PercentOutput"=0, "Position"=1, "Velocity"=2, "Current"=3, "Follower"=5, "MotionProfile"=6, "MotionMagic"=7, "MotionMagicArc"=8, "MotionProfileArc"=10, "Disabled"=15] ("Control Mode")
            w1121 = T6 1 items=["PercentOutput"=0, "Position"=1, "Velocity"=2, "Current"=3, "Follower"=5, "MotionProfile"=6, "MotionMagic"=7, "MotionMagicArc"=8, "MotionProfileArc"=10, "Disabled"=15] ("Control Mode")
            w1119 = T6 1 items=["PercentOutput"=0, "Position"=1, "Velocity"=2, "Current"=3, "Follower"=5, "MotionProfile"=6, "MotionMagic"=7, "MotionMagicArc"=8, "MotionProfileArc"=10, "Disabled"=15] ("Control Mode")
            w1113 = T6 1 items=["PercentOutput"=0, "Position"=1, "Velocity"=2, "Current"=3, "Follower"=5, "MotionProfile"=6, "MotionMagic"=7, "MotionMagicArc"=8, "MotionProfileArc"=10, "Disabled"=15] ("Control Mode")
            # "Turns and Moves the robot based on calculations"
            n783 = local read "ElevatePos"() -> (w1093:dbl)
            n784 = call <vilib>:"WPI_GyroRefNum Registry Get.vi"("refnum name"="Gyro") -> ("GyroDevRef"=w1105:T7)  [unwired: 9 in, 1 out]
            n785 = call "CTRE_Phoenix_MotorControl_RefNumRegistryGet.vi"("refnum name"="Elevator") -> ("PhoenixMotorControlDevRef"=w1092:T10)  [unwired: 9 in, 1 out]
            n786 = call <vilib>:"WPI_GyroGetAngle.vi"("GyroDevRef"=w1105) -> ("Angle"=w1110:dbl)  [unwired: 6 in, 4 out]
            n787 = call "CTRE_Phoenix_MotorControl_Set.vi"("Output"=w1093, "Control Mode"=w1091, "PhoenixMotorControlDevRef"=w1092) -> ()  [unwired: 7 in, 2 out]
            n788 = global read "Robot Global Data.vi" "Gyro Centre"() -> (w1109:dbl)
            n789 = Subtract(x=w1110, y=w1109) -> (x-y=w1108:dbl)
            n790 = Divide(x=w1108, y=360.0) -> (x/y=w1106:dbl)
            n791 = Multiply(x=w1106, y=4096.0) -> (x*y=w1095:dbl)
            n792 = call "CTRE_Phoenix_MotorControl_RefNumRegistryGet.vi"("refnum name"="Turn0") -> ("error out"=w1124:errorcluster, "PhoenixMotorControlDevRef"=w1125:T10)  [unwired: 9 in]
            n793 = call "CTRE_Phoenix_MotorControl_RefNumRegistryGet.vi"("refnum name"="Turn1") -> ("error out"=w1139:errorcluster, "PhoenixMotorControlDevRef"=w1134:T10)  [unwired: 9 in]
            n794 = local read "Direction"() -> (w1101:dbl)
            n795 = local read "Direction 1"() -> (w1096:dbl)
            n796 = call-poly "CTRE_Phoenix_MotorController_Get_Enhanced.vi"("PhoenixMotorControlDevRef"=w1125) -> ("PhoenixMotorControlDevRef"=w1126:T10)  [unwired: 11 in, 3 out]
            n797 = call-poly "CTRE_Phoenix_MotorController_Get_Enhanced.vi"("PhoenixMotorControlDevRef"=w1134) -> ("PhoenixMotorControlDevRef"=w1133:T10)  [unwired: 11 in, 3 out]
            n798 = Add(x=w1095, y=w1101) -> (x+y=w1100:dbl)
            n799 = Add(x=w1095, y=w1096) -> (x+y=w1094:dbl)
            n800 = call "CTRE_Phoenix_MotorControl_Set.vi"("error in (no error)"=w1124, "Output"=w1100, "Control Mode"=w1123, "PhoenixMotorControlDevRef"=w1126) -> ()  [unwired: 6 in, 2 out]
            n801 = call "CTRE_Phoenix_MotorControl_Set.vi"("error in (no error)"=w1139, "Output"=w1094, "Control Mode"=w1113, "PhoenixMotorControlDevRef"=w1133) -> ()  [unwired: 6 in, 2 out]
            n802 = call "CTRE_Phoenix_MotorControl_RefNumRegistryGet.vi"("refnum name"="Turn3") -> ("error out"=w1129:errorcluster, "PhoenixMotorControlDevRef"=w1128:T10)  [unwired: 9 in]
            n803 = call "CTRE_Phoenix_MotorControl_RefNumRegistryGet.vi"("refnum name"="Turn2") -> ("error out"=w1130:errorcluster, "PhoenixMotorControlDevRef"=w1131:T10)  [unwired: 9 in]
            n804 = local read "Direction 2"() -> (w1099:dbl)
            n805 = local read "Direction 3"() -> (w1103:dbl)
            n806 = call-poly "CTRE_Phoenix_MotorController_Get_Enhanced.vi"("PhoenixMotorControlDevRef"=w1128) -> ("PhoenixMotorControlDevRef"=w1127:T10)  [unwired: 11 in, 3 out]
            n807 = call-poly "CTRE_Phoenix_MotorController_Get_Enhanced.vi"("PhoenixMotorControlDevRef"=w1131) -> ("PhoenixMotorControlDevRef"=w1132:T10)  [unwired: 11 in, 3 out]
            n808 = Add(x=w1099, y=w1095) -> (x+y=w1098:dbl)
            n809 = Add(x=w1103, y=w1095) -> (x+y=w1102:dbl)
            n810 = call "CTRE_Phoenix_MotorControl_Set.vi"("error in (no error)"=w1129, "Output"=w1102, "Control Mode"=w1121, "PhoenixMotorControlDevRef"=w1127) -> ()  [unwired: 6 in, 2 out]
            n811 = call "CTRE_Phoenix_MotorControl_Set.vi"("error in (no error)"=w1130, "Output"=w1098, "Control Mode"=w1119, "PhoenixMotorControlDevRef"=w1132) -> ()  [unwired: 6 in, 2 out]
            n812 = local read "speed"() -> (w1140:dbl)
            n813 = call "CTRE_Phoenix_MotorControl_RefNumRegistryGet.vi"("refnum name"="Drive3") -> ("PhoenixMotorControlDevRef"=w1135:T10)  [unwired: 9 in, 1 out]
            n814 = call "CTRE_Phoenix_MotorControl_RefNumRegistryGet.vi"("refnum name"="Drive2") -> ("PhoenixMotorControlDevRef"=w1136:T10)  [unwired: 9 in, 1 out]
            n815 = call "CTRE_Phoenix_MotorControl_RefNumRegistryGet.vi"("refnum name"="Drive1") -> ("PhoenixMotorControlDevRef"=w1137:T10)  [unwired: 9 in, 1 out]
            n816 = call "CTRE_Phoenix_MotorControl_RefNumRegistryGet.vi"("refnum name"="Drive0") -> ("PhoenixMotorControlDevRef"=w1138:T10)  [unwired: 9 in, 1 out]
            n817 = call <vilib>:"WPI_MotorControlSetOutput.vi"("Output"=w1140, "MotorControlDevRef"=w1135) -> ()  [unwired: 7 in, 3 out]
            n818 = call <vilib>:"WPI_MotorControlSetOutput.vi"("Output"=w1140, "MotorControlDevRef"=w1136) -> ()  [unwired: 7 in, 3 out]
            n819 = call <vilib>:"WPI_MotorControlSetOutput.vi"("Output"=w1140, "MotorControlDevRef"=w1137) -> ()  [unwired: 7 in, 3 out]
            n820 = call <vilib>:"WPI_MotorControlSetOutput.vi"("Output"=w1140, "MotorControlDevRef"=w1138) -> ()  [unwired: 7 in, 3 out]
          }
          n821 = stacked-sequence {
            frame #0 {
              n822 = Wait (ms)(milliseconds to wait=u32 750) -> ()  [unwired: 1 out]
            }
            frame #1 {
              w1012 = 0.0 ("Direction")
              n823 = local write "speed"(0.8 ("speed")) -> ()
              n824 = local write "Direction 3"(w1012) -> ()
              n825 = local write "Direction 1"(w1012) -> ()
              n826 = local write "Direction 2"(w1012) -> ()
              n827 = local write "Direction"(w1012) -> ()
              n828 = Wait (ms)(milliseconds to wait=u32 1750) -> ()  [unwired: 1 out]
              n829 = local read "ElevatorPyramid"() -> (w1009:dbl)
              n830 = local write "ElevatePos"(w1009) -> ()
            }
            frame #2 {
              n831 = local read "Scale"() -> (w1013:bool)
              n832 = case shown="False" w1013 {
                frame False {
                  # "2 Scale"
                  n833 = stacked-sequence {
                    frame #0 {
                      n834 = Wait (ms)(milliseconds to wait=u32 1000) -> ()  [unwired: 1 out]
                    }
                    frame #1 {
                      n835 = while {
                        stop <- w1019 stop-if-true
                        n836 = call <vilib>:"WPI_GyroRefNum Registry Get.vi"("refnum name"="Gyro") -> ("GyroDevRef"=w1044:T7)  [unwired: 9 in, 1 out]
                        n837 = call <vilib>:"WPI_GyroGetAngle.vi"("GyroDevRef"=w1044) -> ("Angle"=w1040:dbl)  [unwired: 6 in, 4 out]
                        n838 = global read "Robot Global Data.vi" "Gyro Centre"() -> (w1041:dbl)
                        n839 = Subtract(x=w1040, y=w1041) -> (x-y=w1030:dbl)
                        n840 = Quotient & Remainder(x=w1030, y=360.0) -> (x-y*floor(x/y)=w1028:dbl)  [unwired: 1 out]
                        n841 = Divide(x=w1030, y=360.0) -> (x/y=w1043:dbl)
                        n842 = Multiply(x=w1043, y=4096.0) -> (x*y=w1031:dbl)
                        n843 = Subtract(x=2500.0, y=w1031) -> (x-y=w1038:dbl)
                        n844 = Less Or Equal?(x=w1028, y=330.0) -> (x <= y?=w1025:bool)
                        n845 = Greater Or Equal?(x=w1028, y=300.0) -> (x >= y?=w1024:bool)
                        n846 = local write "Direction"(w1038) -> ()
                        n847 = And(x=w1025, y=w1024) -> (x .and. y?=w1015:bool)
                        n848 = Subtract(x=1500.0, y=w1031) -> (x-y=w1037:dbl)
                        n849 = case shown="False" w1015 {
                          frame False {
                            n850 = local write "speed"(-0.3 ("speed")) -> ()
                          }
                          frame True {
                            n851 = local write "speed"(0.0 ("speed")) -> ()
                          }
                        }
                        n852 = local write "Direction 1"(w1037) -> ()
                        n853 = local read "ElevatorScale"() -> (w1023:dbl)
                        n854 = Subtract(x=500.0, y=w1031) -> (x-y=w1034:dbl)
                        n855 = local write "Direction 2"(w1034) -> ()
                        n856 = local write "ElevatePos"(w1023) -> ()
                        n857 = call "CTRE_Phoenix_MotorControl_RefNumRegistryGet.vi"("refnum name"="Elevator") -> ("error out"=w1020:errorcluster, "PhoenixMotorControlDevRef"=w1021:T10)  [unwired: 9 in]
                        n858 = call-poly "CTRE_Phoenix_MotorController_Get_Enhanced.vi"("PhoenixMotorControlDevRef"=w1021, "error in"=w1020) -> ("Pulse Width Position"=w1018:i32)  [unwired: 8 in, 5 out]
                        n859 = Subtract(x=3500.0, y=w1031) -> (x-y=w1033:dbl)
                        n860 = local write "Direction 3"(w1033) -> ()
                        n861 = Less?(x=w1018, y=-30500) -> (x < y?=w1016:bool)
                        n862 = And(x=w1016, y=w1015) -> (x .and. y?=w1019:bool)
                      }
                    }
                    frame #2 {
                      w1049 = T6 1 items=["PercentOutput"=0, "Position"=1, "Velocity"=2, "Current"=3, "Follower"=5, "MotionProfile"=6, "MotionMagic"=7, "MotionMagicArc"=8, "MotionProfileArc"=10, "Disabled"=15] ("Control Mode")
                      w1054 = 0.0 ("Direction")
                      n863 = call "CTRE_Phoenix_MotorControl_RefNumRegistryGet.vi"("refnum name"="IntakeUp") -> ("PhoenixMotorControlDevRef"=w1052:T10)  [unwired: 9 in, 1 out]
                      n864 = call "CTRE_Phoenix_MotorControl_Set.vi"("Output"=-2000.0, "Control Mode"=w1049, "PhoenixMotorControlDevRef"=w1052) -> ()  [unwired: 7 in, 2 out]
                      n865 = local write "Direction 3"(w1054) -> ()
                      n866 = local write "Direction 2"(w1054) -> ()
                      n867 = local write "Direction 1"(w1054) -> ()
                      n868 = local write "speed"(0.4 ("speed")) -> ()
                      n869 = local write "Direction"(w1054) -> ()
                      n870 = Wait (ms)(milliseconds to wait=u32 1250) -> ()  [unwired: 1 out]
                    }
                    frame #3 {
                      w1060 = T6 0 items=["PercentOutput"=0, "Position"=1, "Velocity"=2, "Current"=3, "Follower"=5, "MotionProfile"=6, "MotionMagic"=7, "MotionMagicArc"=8, "MotionProfileArc"=10, "Disabled"=15] ("Control Mode")
                      w1057 = T6 0 items=["PercentOutput"=0, "Position"=1, "Velocity"=2, "Current"=3, "Follower"=5, "MotionProfile"=6, "MotionMagic"=7, "MotionMagicArc"=8, "MotionProfileArc"=10, "Disabled"=15] ("Control Mode")
                      w1067 = 0.0 ("Direction")
                      n871 = call "CTRE_Phoenix_MotorControl_RefNumRegistryGet.vi"("refnum name"="Intake1") -> ("error out"=w1062:errorcluster, "PhoenixMotorControlDevRef"=w1063:T10)  [unwired: 9 in]
                      n872 = call "CTRE_Phoenix_MotorControl_RefNumRegistryGet.vi"("refnum name"="Intake2") -> ("error out"=w1065:errorcluster, "PhoenixMotorControlDevRef"=w1064:T10)  [unwired: 9 in]
                      n873 = call "CTRE_Phoenix_MotorControl_Set.vi"("error in (no error)"=w1062, "Output"=-1.0, "Control Mode"=w1057, "PhoenixMotorControlDevRef"=w1063) -> ()  [unwired: 6 in, 2 out]
                      n874 = call "CTRE_Phoenix_MotorControl_Set.vi"("error in (no error)"=w1065, "Output"=1.0, "Control Mode"=w1060, "PhoenixMotorControlDevRef"=w1064) -> ()  [unwired: 6 in, 2 out]
                      n875 = local write "Direction 3"(w1067) -> ()
                      n876 = local write "Direction 2"(w1067) -> ()
                      n877 = local write "Direction 1"(w1067) -> ()
                      n878 = local write "speed"(0.0 ("speed")) -> ()
                      n879 = local write "Direction"(w1067) -> ()
                      n880 = Wait (ms)(milliseconds to wait=u32 1000) -> ()  [unwired: 1 out]
                    }
                    frame #4 {
                      w1072 = T6 1 items=["PercentOutput"=0, "Position"=1, "Velocity"=2, "Current"=3, "Follower"=5, "MotionProfile"=6, "MotionMagic"=7, "MotionMagicArc"=8, "MotionProfileArc"=10, "Disabled"=15] ("Control Mode")
                      w1078 = T6 0 items=["PercentOutput"=0, "Position"=1, "Velocity"=2, "Current"=3, "Follower"=5, "MotionProfile"=6, "MotionMagic"=7, "MotionMagicArc"=8, "MotionProfileArc"=10, "Disabled"=15] ("Control Mode")
                      w1075 = T6 0 items=["PercentOutput"=0, "Position"=1, "Velocity"=2, "Current"=3, "Follower"=5, "MotionProfile"=6, "MotionMagic"=7, "MotionMagicArc"=8, "MotionProfileArc"=10, "Disabled"=15] ("Control Mode")
                      w1084 = 2900.0 ("Direction")
                      n881 = call "CTRE_Phoenix_MotorControl_RefNumRegistryGet.vi"("refnum name"="IntakeUp") -> ("PhoenixMotorControlDevRef"=w1069:T10)  [unwired: 9 in, 1 out]
                      n882 = local write "Direction 3"(w1084) -> ()
                      n883 = local write "Direction 2"(w1084) -> ()
                      n884 = local write "Direction 1"(w1084) -> ()
                      n885 = local write "speed"(0.4 ("speed")) -> ()
                      n886 = local write "Direction"(w1084) -> ()
                      n887 = call "CTRE_Phoenix_MotorControl_RefNumRegistryGet.vi"("refnum name"="Intake1") -> ("error out"=w1079:errorcluster, "PhoenixMotorControlDevRef"=w1080:T10)  [unwired: 9 in]
                      n888 = call "CTRE_Phoenix_MotorControl_RefNumRegistryGet.vi"("refnum name"="Intake2") -> ("error out"=w1082:errorcluster, "PhoenixMotorControlDevRef"=w1081:T10)  [unwired: 9 in]
                      n889 = call "CTRE_Phoenix_MotorControl_Set.vi"("Output"=-4500.0, "Control Mode"=w1072, "PhoenixMotorControlDevRef"=w1069) -> ()  [unwired: 7 in, 2 out]
                      n890 = call "CTRE_Phoenix_MotorControl_Set.vi"("error in (no error)"=w1079, "Output"=0.0, "Control Mode"=w1075, "PhoenixMotorControlDevRef"=w1080) -> ()  [unwired: 6 in, 2 out]
                      n891 = call "CTRE_Phoenix_MotorControl_Set.vi"("error in (no error)"=w1082, "Output"=0.0, "Control Mode"=w1078, "PhoenixMotorControlDevRef"=w1081) -> ()  [unwired: 6 in, 2 out]
                      n892 = Wait (ms)(milliseconds to wait=u32 1250) -> ()  [unwired: 1 out]
                    }
                    frame #5 {
                      n893 = local read "ElevatorDown"() -> (w1087:dbl)
                      n894 = local write "speed"(0.0 ("speed")) -> ()
                      n895 = local write "ElevatePos"(w1087) -> ()
                    }
                  }
                }
                frame True {
                  n896 = local read "ElevatorDown"() -> (w1088:dbl)
                  n897 = local write "ElevatePos"(w1088) -> ()
                  n898 = local write "speed"(0.0 ("speed")) -> ()
                }
              }
            }
          }
        }
      }
    }
  }
  "Text" <- ""
  "Current Reading" <- ""
  "x" <- 0.0 ("x")
  "Direction 1" <- 0.0 ("z")
  "Direction 2" <- 0.0 ("z")
  "Direction 3" <- 0.0 ("z")
  "speed" <- 0.0 ("speed")
  "stopped" <- FALSE ("stopped")
  "Direction" <- 0.0 ("Direction")
  "ElevatePos" <- -1500.0 ("ElevatorSwitch")
